vi "FrontPanel.vi"() -> ()   [LabVIEW 2019]
doc: "This VI controls the blindpanel type GHS-2T-1T-700 for a CryoFree DR. Automatization control is embedded in the blindpanel. Keys can be manipulated from within this VI."
uses:
  shared/Inst.FP/Inst.FP.lvclass
  C:/Program Files (x86)/National Instruments/LabVIEW 2019/user.lib/LevyLab/Instrument Framework/SMOs/Instrument/Instrument.lvclass
  C:/Program Files (x86)/National Instruments/LabVIEW 2019/vi.lib/JKI/JKI SMO/SMO/SMO.lvclass
  shared/Inst.FP/Inst.FP.lvclass/Inst.FP.ctl
  shared/Inst.FP/Typedefs/Inst.FP.Push Button--Cluster.ctl
  shared/Inst.FP/Typedefs/Inst.FP.Buttons--Enum.ctl
  <vilib>/Utility/miscctls.llb/LVPointTypeDef.ctl
  ed5445fe-83d3-41b3-b8c0-c155526a2bd6.vi
  <vilib>/JDP Science/JSONtext/JSON text to Variant.vi
  Lib/Lib.llb/ErrCodeStatusLkup.vi
  <vilib>/JDP Science/JSONtext/LVClass Serializer/JSONtext LVClass Serializer.lvclass
  Lib/Lib.llb/Pfeiffer Vacuum.lvlib
  Lib/Lib.llb/MView.lvlib
  Lib/Lib.llb/Busy PopUp.lvlib
  <userlib>/LevyLab/Instrument Framework/SMOs/Instrument/Instrument.lvclass
  <vilib>/JKI/JKI SMO/SMO/SMO.lvclass
panel:
  in  "Inst.FP":refnum<class "Inst.FP.lvclass">
  out "VIRef":T1 {"Array DataType" format="%.0x"; "WaveForm Type" format="%.0x"; "RefNum Type" format="%.0x"; "DataType" format="%.0x"}
  out "ControlNames":string[](array[string])
  in  "Toolbar Panel":enum32{"Page 1", "Page 2"}(tab)
  in  "Load config":bool
  in  "Save config":bool
  in  "Start":bool
  in  "Stop":bool
  out "VI Version":string caption="V"
  out "PT2.Data Array":dbl[](array[numeric])
  in  "Error panel":enum32{"Page 1"}(tab)
  out "PT2.Error":errorcluster
  out "MG.Error":errorcluster
  out "PT1.Error":errorcluster
  out "GHS.Error":errorcluster
  out "PT1.Data Array":dbl[](array[numeric])
  in  "Main Panel":enum32{"Page 1"}(tab)
  out "GHS.P Cluster":T2 {"P1" format="%.1f"; "P2" format="%.1f"; "P3" format="%.1f"; "P4" format="%.1f"; "P5" format="%.1f"; "P6" format="%.1f"; "P7" format="%.1f"; "Flow" format="%#_4f"; "Pstill (P8)" format="%.1e"}
  out "GHS.Alarm?":bool caption="Alarm"
  in  "Main Panel Tabs":T3(tab)
  out "GHS.Layout2.Label1":string
  out "GHS.Layout2.Label2":string
  out "GHS.Layout1.Label1":string
  out "GHS.Layout1.Label2":string
  out "GHS.Mode":u16(ring) items=["AUTO MODE OFF", "START", "CONDENSING 3He", "CONDENSING 4He", "NORMAL CIRCULATION", "RECOVERY OF THE MIXTURE", "RECOVERY: BLOCKAGE OR OVERPRESSURE"]
  out "GHS.Flow":sgl caption="FLOW" format="%#_3f"
  out "GHS.P5":sgl caption="P5"
  out "GHS.P4":sgl caption="P4"
  out "GHS.P3":sgl caption="P3"
  out "GHS.P1":sgl caption="P1"
  out "GHS.P2":sgl caption="P2"
  out "GHS.P7":sgl(slide) caption="3He" min=0 max=2 scale=0.0..2000.0 scale format="%.2f"
  out "GHS.P6":sgl(slide) caption="4He" min=0 max=2 scale=0.0..2000.0 scale format="%.2f"
  out "GHS.Panel ID":string
  in  "GHS Layout Panel":enum32{"OLD", "NEW"}(tab)
  in  "GHS.Layout1.Buttons":T4
  out "GHS.Layout1.LEDs":T5
  in  "GHS.Layout2.Buttons":T4
  out "GHS.Layout2.LEDs":T6
  out "GHS.PC":sgl caption="PC"
  in  "Tab Control 2":enum32{"Plots", "Error Log"}(tab)
  out "PT2 Pressures Plot":cluster{"Time":dbl[], "Value":dbl[]}[](graph)
  out "PT2.Error Log":string[][](table)
  in  "PT2.Start":bool
  in  "PT2.Stop":bool
  in  "PT2.ResetValues":bool
  out "PT2.Error Code":i32 caption="PT Error Code"
  out "PT2.Error Text":string="NO ERROR" caption="PT Error"
  out "PT2.P High":cluster{dbl, dbl, dbl, dbl}(slide) caption="P High" scale=150.0..450.0
  out "PT2.P Low":cluster{dbl, dbl, dbl, dbl}(slide) caption="P Low" scale=0.0..300.0
  out "PT2.P Avg":cluster{"Low":dbl, "High":dbl} caption="P Avg"
  out "PT2.Helium":cluster{dbl, dbl, dbl, dbl}(slide) caption="Helium" scale=0.0..95.0
  out "PT2.Water In":cluster{dbl, dbl, dbl, dbl}(slide) caption="Water In" scale=0.0..35.0
  out "PT2.Water Out":cluster{dbl, dbl, dbl, dbl}(slide) caption="Water Out" scale=0.0..60.0
  out "PT2.State":u16(ring) caption="PT Status" items=["Compressor OFF", "Compressor ON", ""]
  out "PT2.Motor":cluster{dbl, dbl}(slide) caption="Motor" scale=0.0..30.0
  out "PT2.Oil":cluster{dbl, dbl, dbl, dbl}(slide) caption="Oil" scale=0.0..60.0
  out "PT1.P Low":cluster{dbl, dbl, dbl, dbl}(slide) caption="P Low" scale=0.0..300.0
  out "PT1.P High":cluster{dbl, dbl, dbl, dbl}(slide) caption="P High" scale=150.0..450.0
  out "PT1.P Avg":cluster{"Low":dbl, "High":dbl} caption="P Avg"
  out "PT1.Motor":cluster{dbl, dbl}(slide) caption="Motor" scale=0.0..30.0
  out "PT1.Oil":cluster{dbl, dbl, dbl, dbl}(slide) caption="Oil" scale=0.0..60.0
  out "PT1.Helium":cluster{dbl, dbl, dbl, dbl}(slide) caption="Helium" scale=0.0..95.0
  out "PT1.Water Out":cluster{dbl, dbl, dbl, dbl}(slide) caption="Water Out" scale=0.0..60.0
  out "PT1.Water In":cluster{dbl, dbl, dbl, dbl}(slide) caption="Water In" scale=0.0..35.0
  out "PT1.Error Code":i32 caption="PT Error Code"
  out "PT1.Error Text":string="NO ERROR" caption="PT Error"
  in  "PT1.ResetValues":bool
  in  "PT1.Start":bool
  in  "PT1.Stop":bool
  out "PT1.State":u16(ring) caption="PT Status" items=["Compressor OFF", "Compressor ON", ""]
  in  "Tab Control":enum32{"Plots", "Error Log"}(tab)
  out "PT1 Pressures Plot":cluster{"Time":dbl[], "Value":dbl[]}[](graph)
  out "PT1.Error Log":string[][](table)
  out "MG Pressures Plot":cluster{"Time":dbl[], "Value":dbl[]}[](graph)
  out "GHS Pressures Plot":cluster{"Time":dbl[], "Value":dbl[]}[](graph)
  in  "Hide Side Panel":bool
  out "_PT2Port":u16
  out "_PT1Port":u16
  out "_MGPort":refnum<visa-resource-name>="COM4" caption="Port number"
  out "_GHSPort":refnum<visa-resource-name>="COM3" caption="Port number"
  out "_ForceSaveData":bool
  in  "GHS.Button":u8
  out "_SetControl":T7
  in  "S2":enum32{"Page 1"}(tab)
  in  "S2:Reset Error":bool
  in  "S1":enum32{"Page 1"}(tab)
  in  "S1:Reset Error":bool
  out "Curent Log Path":path
  in  "Side Panel":enum32{"Main", "Settings", "Advanced"}(tab)=enum."Settings"
  out "MG.ID String":string caption="ID"
  out "GHS.Response":string caption="Panel response"
  out "MG.Sensors Status":T8={"1"="OK", "2"="OK", "3"="OK", "4"="OK", "5"="OK", "6"="OK"}
  in  "GHS.ADC scaling":T9={"P1"=2500.0, "P2"=2500.0, "P3"=2500.0, "P4"=2500.0, "P5"=2500.0, "P6"=2500.0, "P7"=2500.0, "Flow meter"=682.0, "PC"=10000.0} caption="Front panel ADC scaling factors" {"Flow meter" format="%#.4f"}
  in  "GHS.REC Settings":T10={"P6 low"=20, "P6 high"=1000, "P7 low"=20}
  in  "GHS.NCP5B Settings":cluster{"P6 low":u16}={"P6 low"=20}
  in  "GHS.NCP5 Settings":T10={"P6 low"=20, "P6 high"=1000, "P7 low"=20}
  in  "GHS.S1&2 Settings":cluster{"Enum":enum16{"OFF", "ON"}}
  in  "GHS.P5 Settings":cluster{"P6 low":u16, "P6 high":u16}={"P6 low"=20, "P6 high"=1000}
  out "GHS.REC limits":T11={"P5 warn"=20, "P5 rec"=20, "P5 res"=20}
  out "GHS.NCP5B limits":cluster{"P5 NC4":u16}={"P5 NC4"=20}
  out "GHS.NCP5 limits":T12={"P5 NC1"=20, "P5 NC2"=20, "P5 NC3"=20}
  out "GHS.S1&2 limits":cluster{"S1&S2":enum16{"OFF", "ON"}}
  out "GHS.P5 limits":cluster{"P5 C1":u16, "P5 C2":u16}={"P5 C1"=20, "P5 C2"=20}
  in  "GHS.P6&7 Settings":T13={"P6 low"=20, "P6 high"=1600, "P7 low"=20, "P7 high"=1610}
  out "GHS.P6&7 Limits":T13={"P6 low"=20, "P6 high"=20, "P7 low"=20, "P7 high"=20}
  in  "GHS.Set Values":bool caption="SET VALUES"
  out "MG.Pressures":T14 {"1" format="%-7.2e mbar"; "2" format="%-7.2e mbar"; "3" format="%-7.2e mbar"; "4" format="%-7.2e mbar"; "5" format="%-7.2e mbar"; "6" format="%-7.2e mbar"}
  out "MG.Channel Names":T8={"1"="\"\"", "2"="", "3"="", "4"="", "5"="", "6"=""}
  out "String":string
  in  "Logging Settings":T15={"Plot Data?"=TRUE, "Data Plot Interval"=1.0, "Save Data?"=TRUE, "Data Save Interval"=1.0, "Log Files Folder"=path "C:/LC Data/Data", "Log File Name"="logFP", "Filename Suffix"="_%Y-%m-%d-%H-%M-%S", "New File Interval"=7, "Interval Units"=enum."Days", "Date Format"="%Y-%m-%d %H:%M:%S", "Averages"=4} caption="Data Logging \nOptions" {"Data Save Interval" format="%#_g min"; "Data Plot Interval" format="%#_g min"}
  in  "Hardware Settings":T16={"GHS Port"="COM3", "MG Port"="COM4", "PT1.Enabled?"=FALSE, "MG P8 Channel"=65535, "MG End Recovery?"=FALSE, "PT1 Port"="COM2", "MG Enabled?"=TRUE, "PT1 Address"=16, "S1 Enabled?"=FALSE, "S1 port"="COM2", "S2 Enabled?"=FALSE, "S2 port"="COM2", "Device address S1"=1, "Device address S2"=2, "PT1 Bauds"=115200, "PT2.Enabled?"=FALSE, "PT2 Port"="COM2", "PT2 Address"=16, "PT2 Bauds"=115200, "GHS Bauds"=9600} {"PT2 Address" min=16 max=126 step=1; "MG P8 Channel" items=["Channel 1", "Channel 2", "Channel 3", "Channel 4", "Channel 5", "Channel 6"]; "PT1 Address" min=16 max=126 step=1}
  in  "Automode Settings":T17={"Enable Pressure Check"=FALSE, "Threshold Pressure"=0.0005, "MG Channel"=65535, "Delay Time"=30, "Enable Time Check"=FALSE} {"Delay Time" format="%.0f min"; "MG Channel" items=["Channel 1", "Channel 2", "Channel 3", "Channel 4", "Channel 5", "Channel 6"]; "Threshold Pressure" format="%#_2g mbar"}
  in  "GHS.System Type":enum32{"Wet", "CF"}(radio)=enum."CF" caption="Type"
  in  "GHS.Layout":enum32{"Layout1", "Layout2"}(ring)=enum."Layout2" caption="Panel Layout"
  out "_GHSADCData":dbl[](array[numeric]) caption="Converted ADC Values"
  in  "GHS.Send Command":bool caption="Send"
  out "GHS.Command Response":string
  in  "GHS.Command to Send":string
  out "Automode.Time Reached?":bool
  out "Automode.Pressure Reached?":bool
  out "Automode.Triggered?":bool
  out "Automode.Delay Timer":u32=10 caption="Timer" format="%<%M:%S>t"
  in  "Automode.Start":bool caption="Start"
  out "_VIPath":string caption="VI path"
  out "_GHSRawADCData":i32[](array[numeric]) caption="RAW ADC Values"
  out "MG.Data Array":dbl[](array[numeric]) format="%.3e"
  out "GHS.ADC Data Array":sgl[](array[numeric]) format="%.2f"
  out "GHS.Status Array":u32[](array[numeric])
  # "Error log"
  # "Front panel status"
  # "MaxiGauge status"
  # "Pulse Tube 1 status"
  # "Pulse Tube 2 status"
  # "Leiden Cryogenics"
  # "to \nair"
  # "N.C."
  # "from\novc"
  # "from\nivc"
  # "from still"
  # "to 3He\nin-1"
  # "to 3He\nin-2"
  # "P8"
  # "AUX 1"
  # "BYPASS"
  # "MIXTURE\nCOMPRESSOR"
  # "M2"
  # "P6"
  # "M3"
  # "M1"
  # "AUX PORT-1"
  # "P7"
  # "TRAP"
  # "AUX TRAP"
  # "To \nAir"
  # "From\nIVC"
  # "From Still"
  # "To 3He\nin-1"
  # "To 3He\nin-2"
  # "To \nAir"
  # "N.C."
  # "from\novc"
  # "from\nivc"
  # "from still"
  # "to 3He\nin-1"
  # "to 3He\nin-2"
  # "Leiden Cryogenics"
  # "to \nair"
  # "N.C."
  # "from\novc"
  # "from\nivc"
  # "from still"
  # "to 3He\nin-1"
  # "to 3He\nin-2"
  # "P8"
  # "M2"
  # "P6"
  # "M3"
  # "TRAP"
  # "AUX TRAP"
  # "M1"
  # "AUX PORT-1"
  # "P7"
  # "AUX 1"
  # "To \nAir"
  # "From\nIVC"
  # "From Still"
  # "To 3He\nin-1"
  # "to 3He\nin-1"
  # "To 3He\nin-2"
  # "to \nair"
  # "N.C."
  # "from\novc"
  # "from\nivc"
  # "from still"
  # "to 3He\nin-2"
  # "Pulse Tube 1"
  # "Pulse Tube 2"
  # "Front Panel"
  # "MaxiGauge"
  # "Turbo2 (S2)"
  # "Turbo1 (S1)"
  # "MaxiGauge"
  # "#"
  # "NAME"
  # "PRESSURE"
  # "STATUS"
  # "1"
  # "2"
  # "3"
  # "4"
  # "5"
  # "6"
  # "Automatic mode pressure limits"
  # "Warning: These values influence the operation of the GHS in automatic mode. Please refer to the operation manual and consult with Leiden Cryogenics before changing them."
  # "NAME"
  # "FW"
  # "NEW"
  # "DESCRIPTION"
  # "Stop condensing 4He"
  # "Stop recovering 4He"
  # "Stop condensing 3He"
  # "Stop recovering 3He"
  # "Condensing->open 12"
  # "Condensing->close 9/12"
  # "Condensing->run S1&S2"
  # "NC->open second line"
  # "NC->start MC"
  # "NC->open aux. trap"
  # "NC->stop MC, close 7"
  # "All->P5 alarm"
  # "All->switch to recovery"
  # "All->reset"
  # "Front panel ADC scaling factors"
  # "Data Logging and Plotting"
  # "Front Panel"
  # "MaxiGauge"
  # "Pulse Tube 1"
  # "Pulse Tube 2"
  # "Turbo 1 (S1) (Pfeiffer HiPACE only)"
  # "Turbo2 (S2) (Pfeiffer HiPACE only)"
  # "Automatic condensing"
  # "Send command to Front Panel"
  # "Start condensing when"
  # "and wait"
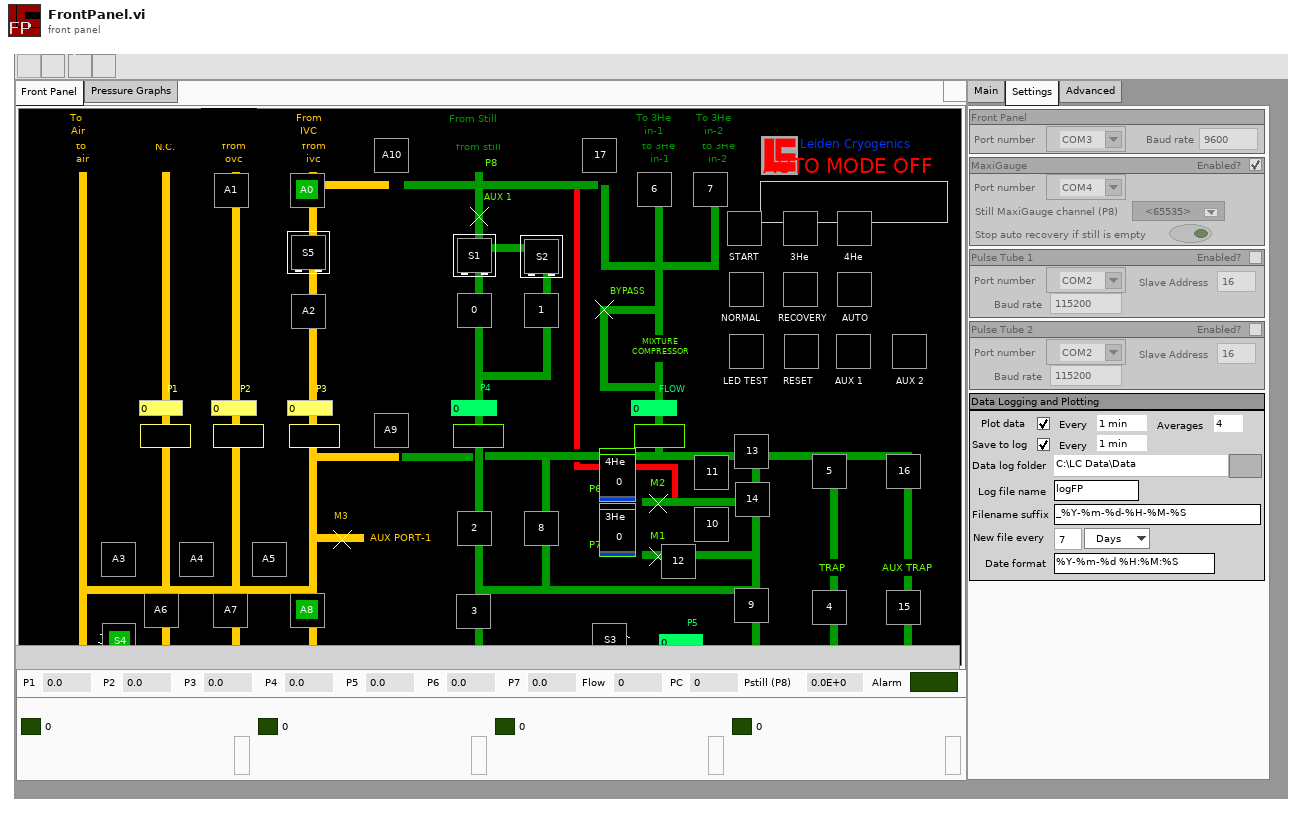
[diagram p1: front panel]
types:
  T1 = cluster{"Control Ref ID":refnum<vi>[], "Full Name":string[], "ClassID":enum16{"<Null>", "1", "2", "Generic", "Decoration", "Text", "Control", "ColorBox", "Boolean", "RefNum", "Variant", "Path", "ListBox", "Table", "Array", "Picture", "ActiveXContainer", "Numeric", "Digital", "NamedNumeric", "ColorRamp", "Slide", "GraphOrChart", "WaveformChart", "WaveformGraph", "IntensityChart", "IntensityGraph", "String", "IOName", "ComboBox", "Cluster", "Panel", "Knob", "NumWithScale", "Ring", "Enum", "GObject", "Plot", "Cursor", "NumericText", "Scale", "ColorScale", "GraphScale", "ColorGraphScale", "TypedRefNum", "OldKnobScale", "MCListbox", "MeasureData", "BVTag", "DAQName", "VISAName", "IVIName", "SlideScale", "TabControl", "Page", "TabArrayTabControl", "ConPane", "57", "58", "59", "60", "61", "62", "63", "64", "SubPanel", "TreeControl", "67", "68", "69", "70", "71", "72", "73", "74", "75", "SplitterBar"}[], "Short Name":string[], "DataType":enum8{"<Null>", "I8", "I16", "I32", "I64", "U8", "U16", "U32", "U64", "SGL", "DBL", "EXT", "CSG", "CDB", "CXT", "0x0F", "0x10", "0x11", "0x12", "0x13", "0x14", "Enum U8", "Enum U16", "Enum U32", "Enum U64", "SGL PQ", "DBL PQ", "EXT PQ", "CSG PQ", "CDB PQ", "CXT PQ", "0x1F", "0x20", "Boolean", "0x22", "0x23", "0x24", "0x25", "0x26", "0x27", "0x28", "0x29", "0x2A", "0x2B", "0x2C", "0x2D", "0x2E", "0x2F", "String", "0x31", "Path", "Pict", "0x34", "0x35", "0x36", "DAQ", "0x38", "0x39", "0x3A", "0x3B", "0x3C", "0x3D", "0x3E", "0x3F", "Array", "0x41", "0x42", "0x43", "0x44", "0x45", "0x46", "0x47", "0x48", "0x49", "0x4A", "0x4B", "0x4C", "0x4D", "0x4E", "0x4F", "Cluster", "0x51", "0x52", "Variant", "Waveform", "0x55", "0x56", "0x57", "0x58", "0x59", "0x5A", "0x5B", "0x5C", "0x5D", "0x5E", "0x5F", "0x60", "0x61", "0x62", "0x63", "0x64", "0x65", "0x66", "0x67", "0x68", "0x69", "0x6A", "0x6B", "0x6C", "0x6D", "0x6E", "0x6F", "Refnum"}[], "RefNum Type":enum8{"Generic", "Datalog File Refnum", "Byte Stream File Refnum", "Device Refnum", "Occurence Refnum", "TCP Connection Refnum", "VISA Refnum (Obsolete)", "Automation Renum", "VI Server Refnum", "Menu Refnum", "IVI Refnum (Obsolete)", "IMAQ Session", "0x0C", "Datasocket Refnum", "VISA Resource", "IVI Logical Name", "UDP Connection Refnum", "Notifier Refnum", "Queue Refnum", "IrDA Refnum", "Hardware Plugin Refnum", "Hardware Plugin Tag Refnum", "DAQmx Refnum", "Event Registration Refnum", ".NET Refnum", "User Event Refnum", "0x1A", "Event Callback", "0x1C", "0x1D", "Only Used Internal to LabVIEW", "Bluetooth", "Data Value References", "RT FIFO", "TDM Streaming"}[], "WaveForm Type":enum8{"<Not a Waveform Type>", "0x01", "Analog 16-bit signed", "Analog Double-Precision", "0x04", "Analog Single Precision", "Timestamp", "Digital Data", "Digital Waveform", "Dynamic Data", "Analog Extended-Precision", "Analog 8-bit unsigned", "Analog 16-bit unsigned", "Analog 32-bit unsigned", "Analog 8-bit signed", "Analog 32-bit signed", "Analog Complex Single-Precision", "Analog Complex Double-Precision", "Analog Complex Extended Precision", "Analog 64-bit signed", "Analog 64-bit unsigned"}[], "Parent":i32[], "Array DataType":enum8{"<Null>", "I8", "I16", "I32", "I64", "U8", "U16", "U32", "U64", "SGL", "DBL", "EXT", "CSG", "CDB", "CXT", "0x0F", "0x10", "0x11", "0x12", "0x13", "0x14", "Enum U8", "Enum U16", "Enum U32", "Enum U64", "SGL PQ", "DBL PQ", "EXT PQ", "CSG PQ", "CDB PQ", "CXT PQ", "0x1F", "0x20", "Boolean", "0x22", "0x23", "0x24", "0x25", "0x26", "0x27", "0x28", "0x29", "0x2A", "0x2B", "0x2C", "0x2D", "0x2E", "0x2F", "String", "0x31", "Path", "Pict", "0x34", "0x35", "0x36", "DAQ", "0x38", "0x39", "0x3A", "0x3B", "0x3C", "0x3D", "0x3E", "0x3F", "Array", "0x41", "0x42", "0x43", "0x44", "0x45", "0x46", "0x47", "0x48", "0x49", "0x4A", "0x4B", "0x4C", "0x4D", "0x4E", "0x4F", "Cluster", "0x51", "0x52", "Variant", "Waveform", "0x55", "0x56", "0x57", "0x58", "0x59", "0x5A", "0x5B", "0x5C", "0x5D", "0x5E", "0x5F", "0x60", "0x61", "0x62", "0x63", "0x64", "0x65", "0x66", "0x67", "0x68", "0x69", "0x6A", "0x6B", "0x6C", "0x6D", "0x6E", "0x6F", "Refnum"}[], "Owning VI":refnum<vi>[], "Active?":bool[]}
  T2 = cluster{"P1":sgl, "P2":sgl, "P3":sgl, "P4":sgl, "P5":sgl, "P6":sgl, "P7":sgl, "Flow":sgl, "PC":sgl, "Pstill (P8)":dbl}
  T3 = enum32{"Front Panel", "PulseTube", "Pressure Graphs"}
  T4 = cluster{"baux2":bool, "bBypass":bool, "b15":bool, "b16":bool, "NC 0":bool, "baux1":bool, "b4":bool, "NC 1":bool, "b5":bool, "breset":bool, "NC 2":bool, "b9":bool, "b14":bool, "NC 3":bool, "b13":bool, "bledtest":bool, "NC 4":bool, "b12":bool, "b10":bool, "NC 5":bool, "b11":bool, "bA0":bool, "NC 9":bool, "b7":bool, "bS3":bool, "NC 12":bool, "b6":bool, "b17":bool, "NC 13":bool, "b8":bool, "b1":bool, "NC 14":bool, "bS2":bool, "b3":bool, "NC 15":bool, "b2":bool, "b0":bool, "NC 16":bool, "bS1":bool, "bA9":bool, "NC 17":bool, "bA8":bool, "bA2":bool, "NC 6":bool, "bs5":bool, "bA10":bool, "NC 7":bool, "bstart":bool, "bA5":bool, "NC 8":bool, "bA7":bool, "bA1":bool, "NC 10":bool, "bauto":bool, "bA4":bool, "NC 11":bool, "bA6":bool, "bS4":bool, "NC 18":bool, "bA3":bool, "b3he":bool, "b4he":bool, "bnorm":bool, "brecov":bool}
  T5 = cluster{"COMPR/AUX 2":bool, "BYPASS":bool, "15":bool, "16":bool, "NC 0":bool, "AUX 1":bool, "4":bool, "NC 1":bool, "5":bool, "RESET":bool, "NC 2":bool, "9":bool, "14":bool, "NC 3":bool, "13":bool, "LED TEST":bool, "NC 4":bool, "12":bool, "10":bool, "NC 5":bool, "11":bool, "A0":bool, "NC 12":bool, "7":bool, "S3":bool, "NC 13":bool, "6":bool, "17":bool, "NC 14":bool, "8":bool, "1":bool, "NC 15":bool, "S2":bool, "3":bool, "NC 16":bool, "2":bool, "0":bool, "NC 17":bool, "S1":bool, "A9":bool, "NC 6":bool, "A8":bool, "A2":bool, "NC 7":bool, "S5":bool, "A10":bool, "NC 8":bool, "START":bool, "A5":bool, "NC 9":bool, "A7":bool, "A1":bool, "NC 10":bool, "AUTO":bool, "A4":bool, "NC 11":bool, "A6":bool, "S4":bool, "NC 18":bool, "A3":bool, "3He":bool, "4He":bool, "NORMAL":bool, "RECOVERY":bool, "PT STATUS":bool}
  T6 = cluster{"COMPR/AUX 2":bool, "BYPASS":bool, "15":bool, "16":bool, "AUX 1":bool, "AUX 1":bool, "4":bool, "AUX 2":bool, "5":bool, "RESET":bool, "AUX 3":bool, "9":bool, "14":bool, "NC 3":bool, "13":bool, "LED TEST":bool, "NC 4":bool, "12":bool, "10":bool, "NC 5":bool, "11":bool, "A0":bool, "NC 12":bool, "7":bool, "S3":bool, "NC 13":bool, "6":bool, "17":bool, "NC 14":bool, "8":bool, "1":bool, "NC 15":bool, "S2":bool, "3":bool, "NC 16":bool, "2":bool, "0":bool, "NC 17":bool, "S1":bool, "A9":bool, "NC 6":bool, "A8":bool, "A2":bool, "NC 7":bool, "S5":bool, "A10":bool, "NC 8":bool, "START":bool, "A5":bool, "NC 9":bool, "A7":bool, "A1":bool, "NC 10":bool, "AUTO":bool, "A4":bool, "NC 11":bool, "A6":bool, "S4":bool, "NC 18":bool, "A3":bool, "3He":bool, "4He":bool, "NORMAL":bool, "RECOVERY":bool, "PT STATUS":bool}
  T7 = cluster{"Name":string, "Scalar":string, "Array":string[][]}
  T8 = cluster{"1":string, "2":string, "3":string, "4":string, "5":string, "6":string}
  T9 = cluster{"P1":dbl, "P2":dbl, "P3":dbl, "P4":dbl, "P5":dbl, "P6":dbl, "P7":dbl, "Flow meter":dbl, "PC":dbl}
  T10 = cluster{"P6 low":u16, "P6 high":u16, "P7 low":u16}
  T11 = cluster{"P5 warn":u16, "P5 rec":u16, "P5 res":u16}
  T12 = cluster{"P5 NC1":u16, "P5 NC2":u16, "P5 NC3":u16}
  T13 = cluster{"P6 low":u16, "P6 high":u16, "P7 low":u16, "P7 high":u16}
  T14 = cluster{"1":dbl, "2":dbl, "3":dbl, "4":dbl, "5":dbl, "6":dbl}
  T15 = cluster{"Plot Data?":bool, "Data Plot Interval":dbl, "Save Data?":bool, "Data Save Interval":dbl, "Log Files Folder":path, "Log File Name":string, "Filename Suffix":string, "New File Interval":u32, "Interval Units":enum16{"Minutes", "Hours", "Days"}, "Date Format":string, "Averages":i32}
  T16 = cluster{"GHS Port":refnum<visa-resource-name>, "MG Port":refnum<visa-resource-name>, "PT1.Enabled?":bool, "MG P8 Channel":u16, "MG End Recovery?":bool, "PT1 Port":refnum<visa-resource-name>, "MG Enabled?":bool, "PT1 Address":u8, "S1 Enabled?":bool, "S1 port":refnum<visa-resource-name>, "S2 Enabled?":bool, "S2 port":refnum<visa-resource-name>, "Device address S1":u8, "Device address S2":u8, "PT1 Bauds":u32, "PT2.Enabled?":bool, "PT2 Port":refnum<visa-resource-name>, "PT2 Address":u8, "PT2 Bauds":u32, "GHS Bauds":u32}
  T17 = cluster{"Enable Pressure Check":bool, "Threshold Pressure":dbl, "MG Channel":u16, "Delay Time":u32, "Enable Time Check":bool}
  T18 = typedef "Inst.FP.lvclass/PublicEvents--Cluster.ctl" = cluster{"MessageFromProcess":refnum<user-event>}
  T19 = cluster{"error":bool, "code":i32, "source":string}
  T20 = cluster{"Dict. Var":u16, "Description":string, "Values":i32[]}[]
  T21 = cluster{"[3]":dbl, "[3]":dbl, "[3]":dbl, "Values[3] 2":dbl}
  T22 = cluster{"[1]":dbl, "[1]":dbl, "[1]":dbl, "Values[1] 2":dbl}
  T23 = cluster{"Values[0]":dbl, "Values[0]":dbl, "Values[0]":dbl, "Values[0] 2":dbl}
  T24 = cluster{"error":bool, "code":i32, "error source":string}
  T25 = cluster{"sensor status info[0]":string, "sensor status info[1]":string, "sensor status info[2]":string, "sensor status info[3]":string, "sensor status info[4]":string, "sensor status info[5]":string}
  T26 = cluster{"Filterred[0]":dbl, "Filterred[1]":dbl, "Filterred[2]":dbl, "Filterred[3]":dbl, "Filterred[4]":dbl, "Filterred[5]":dbl}
  T27 = typedef "Inst.FP.lvclass/Inst.FP.Push Button--Cluster.ctl" = cluster{"Button":T28}
  T28 = typedef "Inst.FP.lvclass/Inst.FP.Buttons--Enum.ctl" = enum16{"Start", "3He", "4He", "Normal", "Recovery", "Auto", "LED Test", "Reset"}
  T29 = cluster{"GHS.ADC Data Array[0]":sgl, "GHS.ADC Data Array[1]":sgl, "GHS.ADC Data Array[2]":sgl, "GHS.ADC Data Array[3]":sgl, "GHS.ADC Data Array[4]":sgl, "GHS.ADC Data Array[5]":sgl, "GHS.ADC Data Array[6]":sgl, "GHS.ADC Data Array[7]":sgl, "GHS.ADC Data Array[8]":sgl}
  T30 = cluster{"GHS.ADC Data Array[0]":sgl, "GHS.ADC Data Array[1]":sgl, "GHS.ADC Data Array[2]":sgl, "GHS.ADC Data Array[3]":sgl, "GHS.ADC Data Array[4]":sgl, "GHS.ADC Data Array[5]":sgl, "GHS.ADC Data Array[6]":sgl, "GHS.ADC Data Array[7]":sgl, "GHS.ADC Data Array[8]":sgl, dbl}
  T31 = enum32{"Page Enabled", "Page Disabled", "Page Disabled & Grayed"}
  T32 = enum32{"invalid app kind", "Development System", "Run Time System", "Student Edition", "Embedded LabVIEW", "Evaluation", "Custom"}
  T33 = cluster{"array of 4 x 16 bit unsigned[0]":u16, "array of 4 x 16 bit unsigned[1]":u16, "array of 4 x 16 bit unsigned[2]":u16, "array of 4 x 16 bit unsigned[3]":u16}
  T34 = cluster{"array of 2 x 16 bit unsigned[0]":u16, "array of 2 x 16 bit unsigned[1]":u16}
  T35 = cluster{"array of 3 x 16 bit unsigned[0]":u16, "array of 3 x 16 bit unsigned[1]":u16, "array of 3 x 16 bit unsigned[2]":u16}
  T36 = cluster{"Array[0]":string, "Array[1]":string, "Array[2]":string, "Array[3]":string, "Array[4]":string, "Array[5]":string}
  T37 = typedef "LVPointTypeDef.ctl" = cluster{"Horizontal":i16, "Vertical":i16}
  T38 = typedef "LVRectTypeDef.ctl" = cluster{"Left":i16, "Top":i16, "Right":i16, "Bottom":i16}
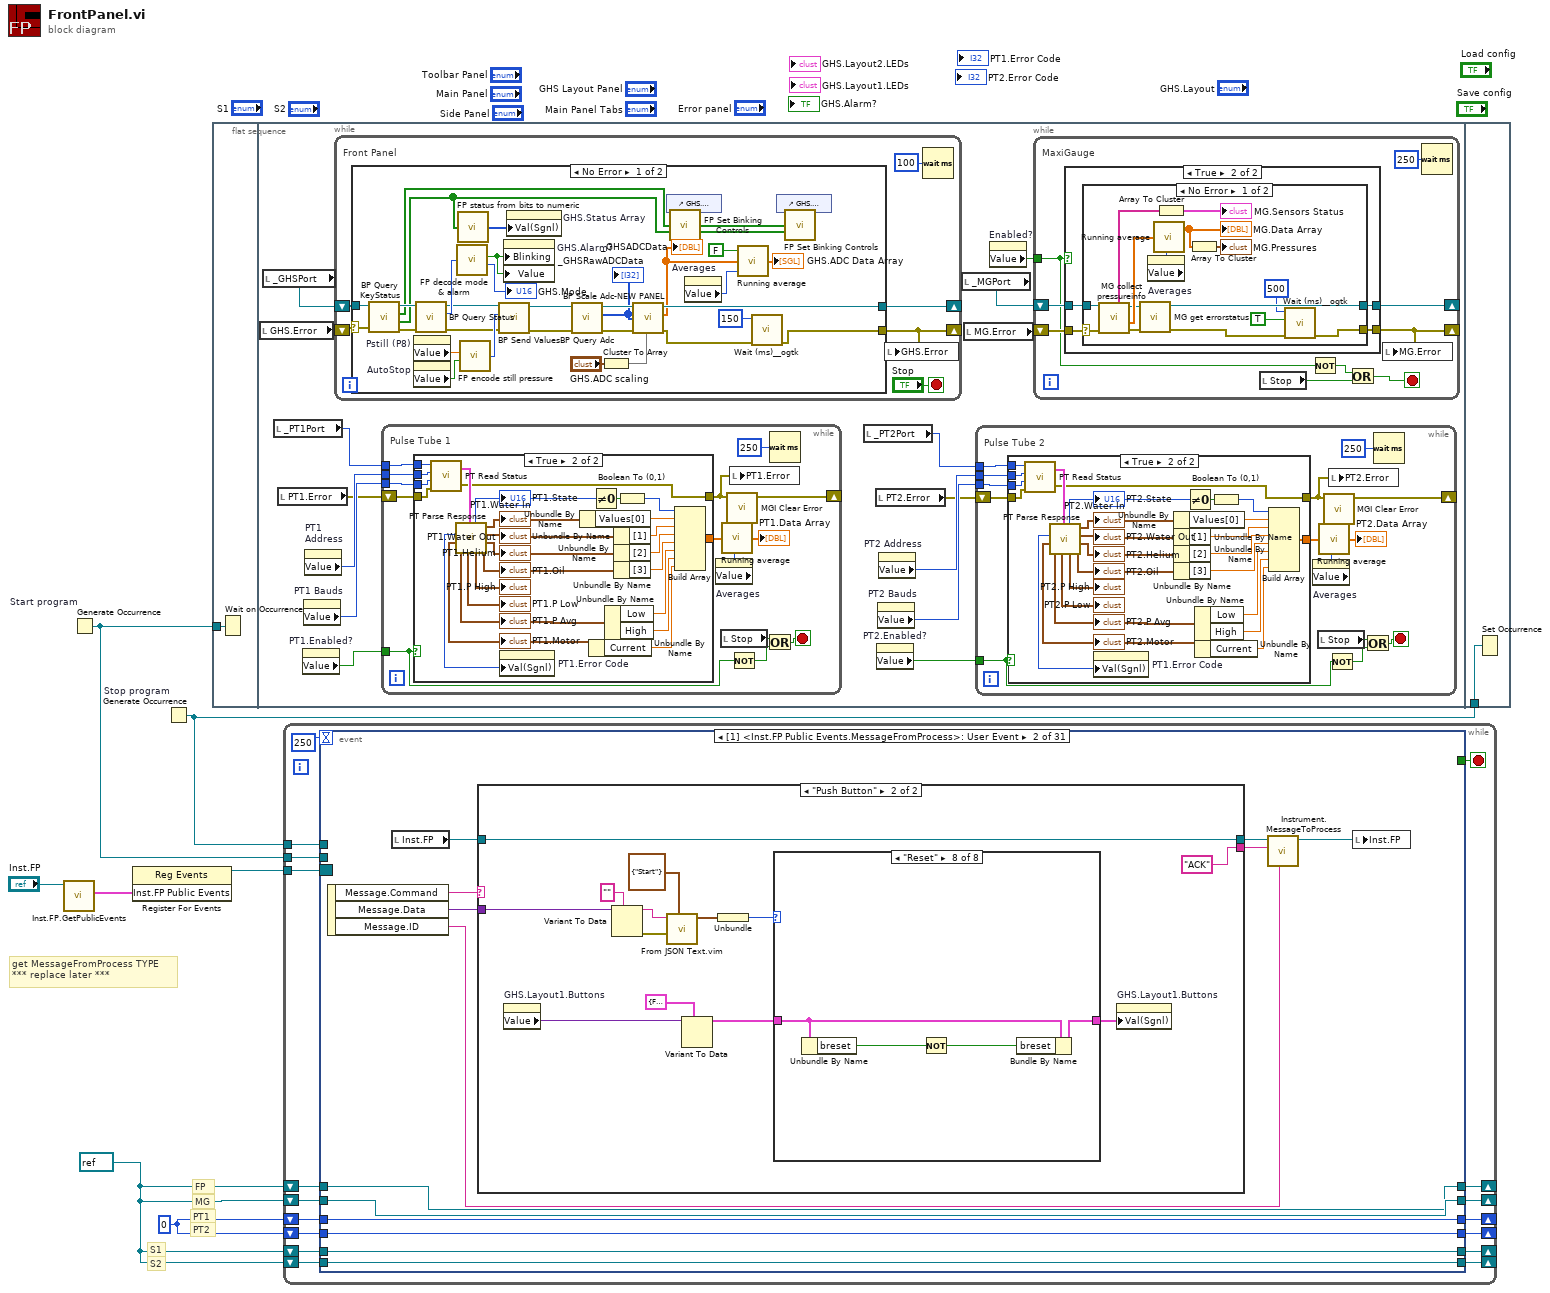
[diagram p0: block diagram]
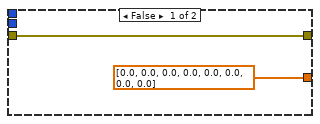
[diagram p2: hidden frame]
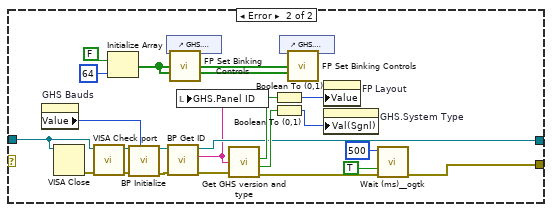
[diagram p3: hidden frame]
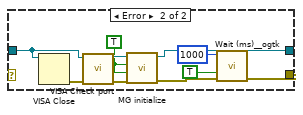
[diagram p5: hidden frame]
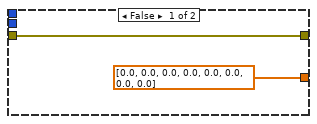
[diagram p6: hidden frame]
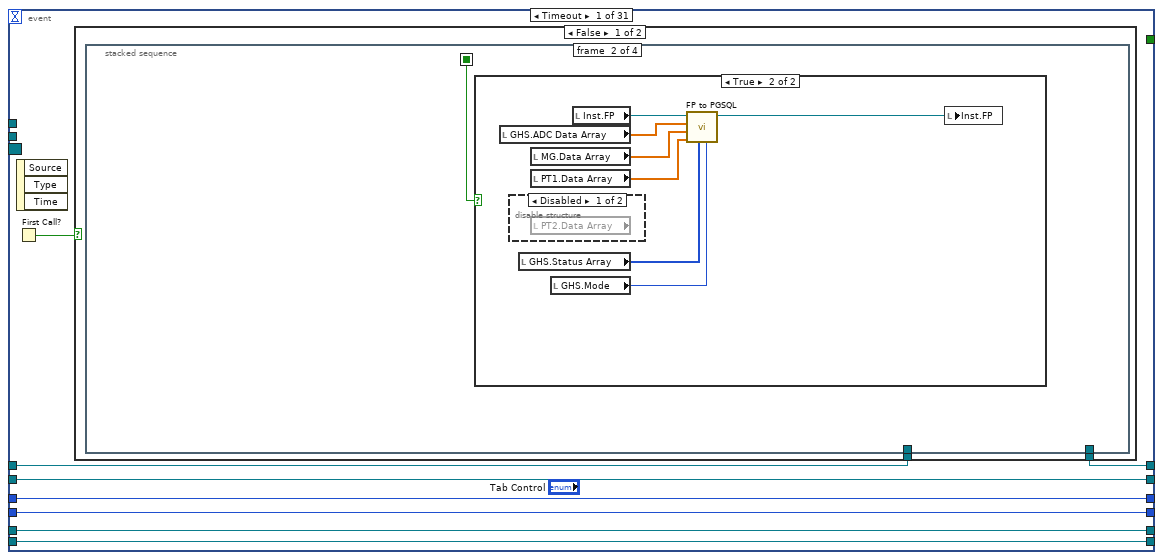
[diagram p7: hidden frame]
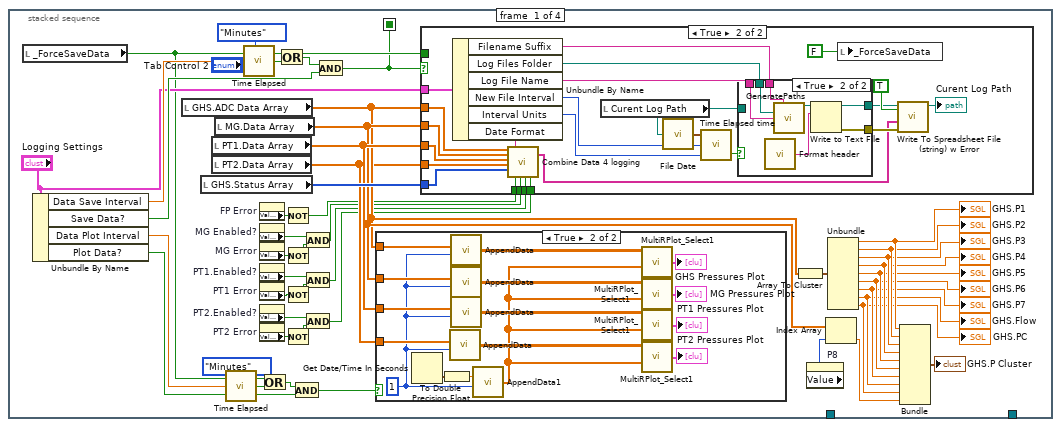
[diagram p8: hidden frame]
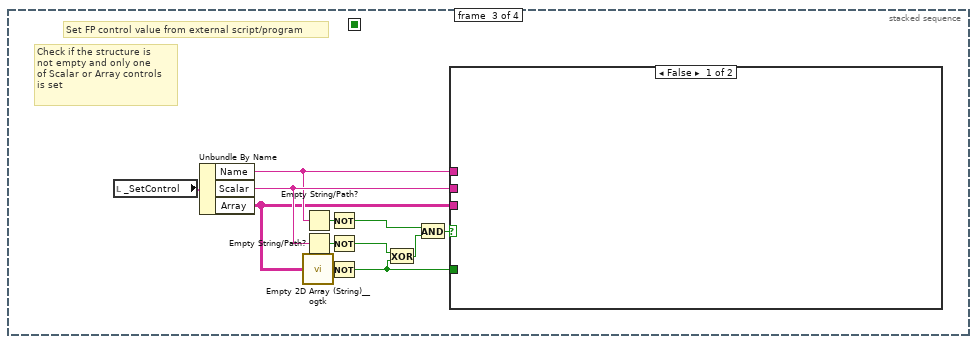
[diagram p14: hidden frame]
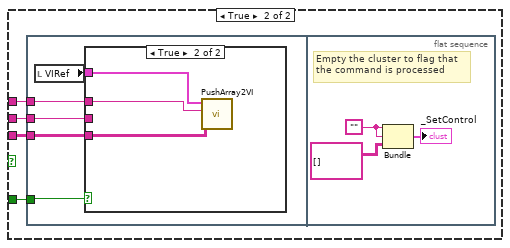
[diagram p15: hidden frame]
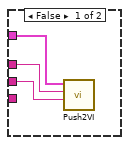
[diagram p16: hidden frame]
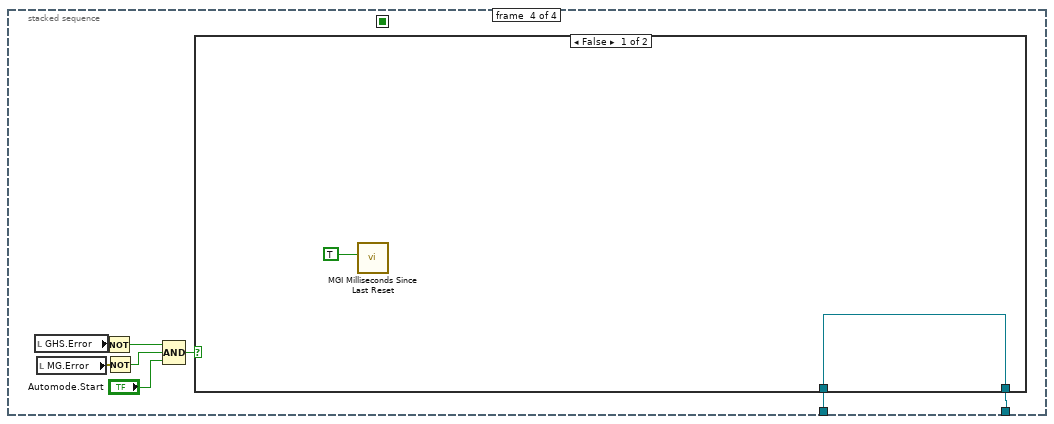
[diagram p17: hidden frame]
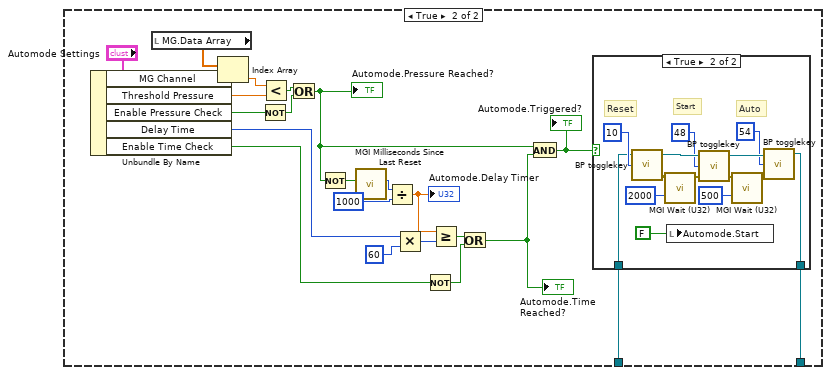
[diagram p18: hidden frame]
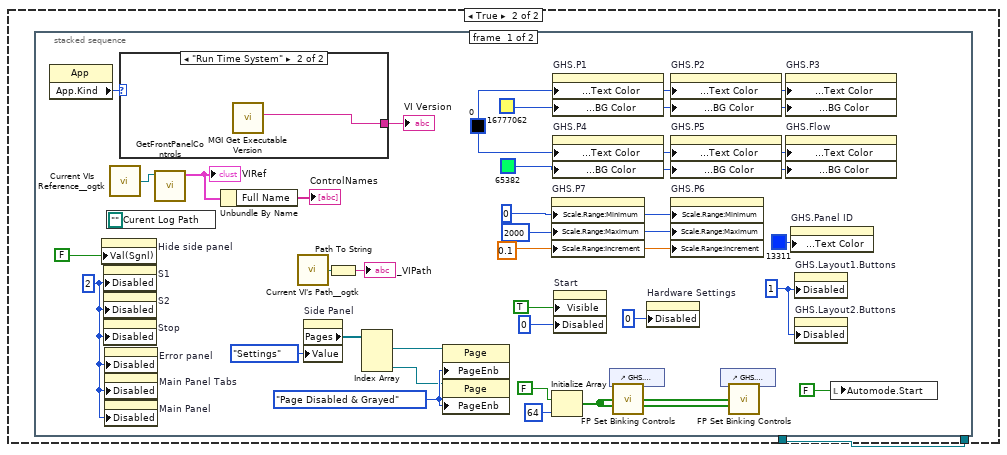
[diagram p20: hidden frame]
diagram:
  w4 = u8 0 ("x+1")
  w5 = refnum<visa-resource-name> refnum ("PT port")
  # "get MessageFromProcess TYPE\n*** replace later ***"
  # "S2"
  # "S1"
  # "MG"
  # "PT1"
  # "PT2"
  # "FP"
  n1 = call "Inst.FP.GetPublicEvents.vi"("Inst.FP in"="Inst.FP") -> ("Inst.FP Public Events"=w2:T18)  [unwired: 8 in, 2 out]
  n2 = Generate Occurrence "Start program"() -> (w7:refnum<k4>)
  n3 = register-events(w2) -> (reference out=w3:refnum<event-registration>)  [unwired: 2 in, 1 out]
  n4 = Generate Occurrence "Stop program"() -> (w6:refnum<k4>)
  n5 = flat-sequence {
    tunnel: w7 -> [w8]
    tunnel: w6 -> [w207]
    frame #0 {
      n6 = Wait on Occurrence(2:w8) -> ()  [unwired: 2 in, 1 out]
    }
    frame #1 {
      n7 = local read "GHS.Error"() -> (w19:errorcluster)
      n8 = local read "_GHSPort"() -> (w14:refnum<visa-resource-name>)
      n9 = local read "_PT1Port"() -> (w10:u16)
      n10 = local read "PT1.Error"() -> (w11:errorcluster)
      n11 = property on="PT1.Enabled?" class="Bool (strict)"() -> ("Value"=w22:bool)  [unwired: 2 in, 2 out]
      n12 = property on="PT1 Bauds" class="DigNum (strict)"() -> ("Value"=w20:u32)  [unwired: 2 in, 2 out]
      n13 = property on="PT1 \nAddress" class="DigNum (strict)"() -> ("Value"=w23:u8)  [unwired: 2 in, 2 out]
      n14 = while {
        shift-right: [w69] -> _
        shift-left: w19 -> [w70]
        shift-right: [w67] -> _
        shift-left: w14 -> [w68]
        stop <- "Stop" stop-if-true
        # "Front Panel"
        n15 = case shown="No Error" w70 {
          selector: w70 -> [w100 _]
          tunnel: [w81 w114] -> w67
          tunnel: [w79 w112] -> w69
          tunnel: w68 -> [w101 w115]
          frame No Error {
            n16 = call "BP Query KeyStatus.vi"("error in"=w100, "FrontPanel port"=w101) -> ("error out"=w89:T19, "Button states"=w72:bool[], "Blinking States"=w73:bool[], "FrontPanel port"=w90:refnum<visa-resource-name>)  [unwired: 2 in]
            n17 = property on="Pstill (P8)" class="DigNum (strict)"() -> ("Value"=w91:dbl)  [unwired: 2 in, 2 out]
            n18 = property on="AutoStop" class="Bool (strict)"() -> ("Value"=w92:bool)  [unwired: 2 in, 2 out]
            n19 = call "BP Query Status.vi"("error in"=w89, "FrontPanel port"=w90) -> ("error out"=w94:T19, "status word (32 bit unsigned)"=w97:u32, "FrontPanel port"=w95:refnum<visa-resource-name>)  [unwired: 3 in]
            n20 = call "FP decode mode & alarm.vi"("status word (32 bit unsigned)"=w97) -> ("Boolean"=w93:bool, "Numeric"=→"GHS.Mode":u32)  [unwired: 4 in]
            n21 = call "FP status from bits to numeric.vi"("FP Status bits"=w72) -> ("FP status number"=w99:u32[])  [unwired: 4 in]
            n22 = call "FP encode still pressure.vi"("Value 2"=w92, "Value"=w91) -> ("Numeric"=w96:u16)  [unwired: 4 in]
            n23 = call "BP Send Values.vi"("error in"=w94, "value to send"=w96, "FrontPanel port"=w95) -> ("error out"=w83:T19, "FrontPanel port"=w84:refnum<visa-resource-name>)  [unwired: 3 in]
            n24 = property on="GHS.Alarm?" class="Bool (strict)"("Blinking"=w93, "Value"=w93) -> ()  [unwired: 2 in, 2 out]
            n25 = property on="GHS.Status Array" class="Arr (strict)"("Val(Sgnl)"=w99) -> ()  [unwired: 2 in, 2 out]
            n26 = call "BP Query Adc.vi"("error in"=w83, "FrontPanel port"=w84) -> ("error out"=w80:T19, "array of 9 x 16 bit signed"=w75:i32[], "FrontPanel port"=w81:refnum<visa-resource-name>)  [unwired: 3 in]
            "_GHSRawADCData" <- w75
            n27 = Cluster To Array(cluster="GHS.ADC scaling") -> (array=w82:dbl[])
            n28 = call "BP Scale Adc-NEW PANEL.vi"("input array scaling factors,8(9) x 16 bit uint"=w82, "input array 8(9) x 16bit uint"=w75) -> ("output array 8(9) x single prec. incl flow"=w74:sgl[])  [unwired: 4 in, 1 out]
            "_GHSADCData" <- w74
            n29 = control-ref of="GHS.Layout1.LEDs"() -> (w77:refnum<vi>)
            n30 = call "FP Set Binking Controls.vi"("Cluster in"=w77, "Array of blinking states"=w73, "Array of relais states"=w72) -> ()  [unwired: 13 in]
            n31 = property on="Averages" class="DigNum (strict)"() -> ("Value"=w88:i32)  [unwired: 2 in, 2 out]
            n32 = call "Running average.vi"("Window Size"=w88, "New values"=w74, "Filter Zeroes? (T)"=FALSE) -> ("Filterred"=→"GHS.ADC Data Array":dbl[])  [unwired: 1 in]
            n33 = call <userlib>:"Wait (ms)__ogtk.vi"("error in (no error)"=w80, "milliseconds to wait"=u32 150) -> ("error out"=w79:errorcluster)  [unwired: 8 in, 1 out]
            n34 = control-ref of="GHS.Layout2.LEDs"() -> (w76:refnum<vi>)
            n35 = call "FP Set Binking Controls.vi"("Cluster in"=w76, "Array of blinking states"=w73, "Array of relais states"=w72) -> ()  [unwired: 13 in]
          }
          frame Error {
            n36 = property on="GHS Bauds" class="DigNum (strict)"() -> ("Value"=w107:u32)  [unwired: 2 in, 2 out]
            n37 = VISA Close(VISA resource name=w115) -> (error out=w124:errorcluster)  [unwired: 1 in]
            n38 = call "VISA Check port.vi"("error in (no error)"=w124, "VISA Resource Name in"=w115) -> ("error out"=w123:errorcluster, "VISA Resource Name out"=w122:refnum<visa-resource-name>)  [unwired: 8 in]
            n39 = Initialize Array(FALSE, 64 ("dimension size")) -> (w102:bool[])
            n40 = call "BP Initialize.vi"("FP baud rate"=w107, "error in (no error)"=w123, "FrontPanel port"=w122) -> ("error out"=w121:errorcluster, "FrontPanel port"=w120:refnum<visa-resource-name>)  [unwired: 4 in]
            n41 = control-ref of="GHS.Layout1.LEDs"() -> (w104:refnum<vi>)
            n42 = call "BP Get ID.vi"("error in (no error)"=w121, "FrontPanel port"=w120) -> ("error out"=w109:errorcluster, "Device ID string"=w113:string, "FrontPanel port"=w114:refnum<visa-resource-name>)  [unwired: 6 in, 1 out]
            n43 = call "FP Set Binking Controls.vi"("Cluster in"=w104, "Array of blinking states"=w102, "Array of relais states"=w102) -> ()  [unwired: 13 in]
            n44 = local write "GHS.Panel ID"(w113) -> ()
            n45 = call "Get GHS version and type.vi"("ID string"=w113, "error in (no error)"=w109) -> ("Panel Version"=w116:bool, "System Type"=w118:bool, "error out"=w108:errorcluster)  [unwired: 4 in]
            n46 = Boolean To (0,1)(Boolean=w116) -> (0, 1=w117:i16)
            n47 = Boolean To (0,1)(Boolean=w118) -> (0, 1=w119:i16)
            n48 = control-ref of="GHS.Layout2.LEDs"() -> (w103:refnum<vi>)
            n49 = call "FP Set Binking Controls.vi"("Cluster in"=w103, "Array of blinking states"=w102, "Array of relais states"=w102) -> ()  [unwired: 13 in]
            n50 = property on="FP Layout" class="TabCtl (strict)"("Value"=w117) -> ()  [unwired: 2 in, 2 out]
            n51 = property on="GHS.System Type" class="RadioBtnsControl (strict)"("Val(Sgnl)"=w119) -> ()  [unwired: 2 in, 2 out]
            n52 = call <userlib>:"Wait (ms)__ogtk.vi"("error in (no error)"=w108, "Wait on Error (FALSE)"=TRUE, "milliseconds to wait"=u32 500) -> ("error out"=w112:errorcluster)  [unwired: 7 in, 1 out]
          }
        }
        n53 = local write "GHS.Error"(w69) -> ()
        n54 = Wait (ms)(milliseconds to wait=u32 100) -> ()  [unwired: 1 out]
      }
      n55 = while {
        tunnel: w10 -> [w177]
        tunnel: w23 -> [w176]
        tunnel: w22 -> [w167]
        tunnel: w20 -> [w173]
        shift-right: [w166] -> _
        shift-left: w11 -> [w172]
        stop <- w170 stop-if-true
        # "Pulse Tube 1"
        n56 = case shown="True" w167 {
          tunnel: [dbl[] [0.0, 0.0, 0.0, 0.0, 0.0, 0.0, 0.0, 0.0] w194] -> w178
          tunnel: w177 -> [_ w193]
          tunnel: w172 -> [w179 w192]
          tunnel: w176 -> [_ w191]
          tunnel: w173 -> [_ w186]
          tunnel: [w179 w185] -> w165
          frame False {
          }
          frame True {
            n57 = call "PT Read Status.vi"("error in (no error)"=w192, "Baud"=w186, "Slave Address"=w191, "Com Port #"=w193) -> ("error out"=w185:errorcluster, "Response"=w195:T20)
            n58 = call "PT Parse Response.vi"("Response"=w195) -> ("Oil temp"=w200:T21, "He temp"=w199:cluster{"[2]":dbl, "[2]":dbl, "[2]":dbl, dbl}, "Out water temp"=w198:T22, "In water temp"=w197:T23, "P_high"=→"PT1.P High":cluster{"[0]":dbl, "[0]":dbl, "[0]":dbl, dbl}, "Numeric"=w204:i32, "P_low"=→"PT1.P Low":cluster{"[1]":dbl, "[1]":dbl, "[1]":dbl, dbl}, "Average pressure"=w190:cluster{"Low":dbl, "High":dbl}, "Current"=w184:cluster{"Current":dbl, "Threshold":dbl}, "PT Error"=w196:i32)  [unwired: 1 in]
            "PT1.Oil" <- w200
            "PT1.Motor" <- w184
            "PT1.State" <- w204
            "PT1.Water Out" <- w198
            "PT1.Water In" <- w197
            "PT1.Helium" <- w199
            "PT1.P Avg" <- w190
            n59 = property on="PT1.Error Code" class="DigNum (strict)"("Val(Sgnl)"=w196) -> ()  [unwired: 2 in, 2 out]
            n60 = Unbundle By Name(w197) -> ("Values[0]"=w187:dbl)
            n61 = Unbundle By Name(w184) -> ("Current"=w183:dbl)
            n62 = Not Equal To 0?(x=w204) -> (x != 0?=w205:bool)
            n63 = Unbundle By Name(w190) -> ("Low"=w189:dbl, "High"=w188:dbl)
            n64 = Unbundle By Name(w198) -> ("[1]"=w203:dbl)
            n65 = Unbundle By Name(w199) -> ("[2]"=w202:dbl)
            n66 = Unbundle By Name(w200) -> ("[3]"=w201:dbl)
            n67 = Boolean To (0,1)(Boolean=w205) -> (0, 1=w206:i16)
            n68 = Build Array(w206, w187, w203, w202, w201, w189, w188, w183) -> (w194:dbl[])
          }
        }
        n69 = property on="Averages" class="DigNum (strict)"() -> ("Value"=w175:i32)  [unwired: 2 in, 2 out]
        n70 = local read "Stop"() -> (w169:bool)
        n71 = call "Running average.vi"("Window Size"=w175, "New values"=w178) -> ("Filterred"=→"PT1.Data Array":dbl[])  [unwired: 2 in]
        n72 = call <userlib>:"MGI Clear Error.vi"("Error In"=w165) -> ("Error Out"=w166:errorcluster)  [unwired: 6 in]
        n73 = Not(x=w167) -> (.not. x?=w168:bool)
        n74 = local write "PT1.Error"(w165) -> ()
        n75 = Or(x=w169, y=w168) -> (x .or. y?=w170:bool)
        n76 = Wait (ms)(milliseconds to wait=u32 250) -> ()  [unwired: 1 out]
      }
      n77 = local read "_PT2Port"() -> (w9:u16)
      n78 = local read "PT2.Error"() -> (w12:errorcluster)
      n79 = property on="PT2.Enabled?" class="Bool (strict)"() -> ("Value"=w16:bool)  [unwired: 2 in, 2 out]
      n80 = property on="PT2 Bauds" class="DigNum (strict)"() -> ("Value"=w15:u32)  [unwired: 2 in, 2 out]
      n81 = property on="PT2 Address" class="DigNum (strict)"() -> ("Value"=w17:u8)  [unwired: 2 in, 2 out]
      n82 = local read "_MGPort"() -> (w13:refnum<visa-resource-name>)
      n83 = local read "MG.Error"() -> (w18:errorcluster)
      n84 = while {
        tunnel: w9 -> [w36]
        tunnel: w17 -> [w35]
        tunnel: w16 -> [w26]
        tunnel: w15 -> [w32]
        shift-right: [w25] -> _
        shift-left: w12 -> [w31]
        stop <- w29 stop-if-true
        # "Pulse Tube 2"
        n85 = case shown="True" w26 {
          tunnel: [dbl[] [0.0, 0.0, 0.0, 0.0, 0.0, 0.0, 0.0, 0.0] w53] -> w37
          tunnel: w36 -> [_ w52]
          tunnel: w31 -> [w38 w51]
          tunnel: w35 -> [_ w50]
          tunnel: w32 -> [_ w45]
          tunnel: [w38 w44] -> w24
          frame False {
          }
          frame True {
            n86 = call "PT Read Status.vi"("error in (no error)"=w51, "Baud"=w45, "Slave Address"=w50, "Com Port #"=w52) -> ("error out"=w44:errorcluster, "Response"=w54:T20)
            n87 = call "PT Parse Response.vi"("Response"=w54) -> ("Oil temp"=w59:T21, "He temp"=w58:cluster{"[2]":dbl, "[2]":dbl, "[2]":dbl, dbl}, "Out water temp"=w57:T22, "In water temp"=w56:T23, "P_high"=→"PT2.P High":cluster{"[0]":dbl, "[0]":dbl, "[0]":dbl, dbl}, "Numeric"=w63:i32, "P_low"=→"PT2.P Low":cluster{"[1]":dbl, "[1]":dbl, "[1]":dbl, dbl}, "Average pressure"=w49:cluster{"Low":dbl, "High":dbl}, "Current"=w43:cluster{"Current":dbl, "Threshold":dbl}, "PT Error"=w55:i32)  [unwired: 1 in]
            "PT2.Oil" <- w59
            "PT2.Motor" <- w43
            "PT2.State" <- w63
            "PT2.Water Out" <- w57
            "PT2.Water In" <- w56
            "PT2.Helium" <- w58
            "PT2.P Avg" <- w49
            n88 = property on="PT1.Error Code" class="DigNum (strict)"("Val(Sgnl)"=w55) -> ()  [unwired: 2 in, 2 out]
            n89 = Unbundle By Name(w56) -> ("Values[0]"=w46:dbl)
            n90 = Unbundle By Name(w57) -> ("[1]"=w62:dbl)
            n91 = Unbundle By Name(w58) -> ("[2]"=w61:dbl)
            n92 = Unbundle By Name(w59) -> ("[3]"=w60:dbl)
            n93 = Not Equal To 0?(x=w63) -> (x != 0?=w64:bool)
            n94 = Unbundle By Name(w49) -> ("Low"=w48:dbl, "High"=w47:dbl)
            n95 = Unbundle By Name(w43) -> ("Current"=w42:dbl)
            n96 = Boolean To (0,1)(Boolean=w64) -> (0, 1=w65:i16)
            n97 = Build Array(w65, w46, w62, w61, w60, w48, w47, w42) -> (w53:dbl[])
          }
        }
        n98 = property on="Averages" class="DigNum (strict)"() -> ("Value"=w34:i32)  [unwired: 2 in, 2 out]
        n99 = local read "Stop"() -> (w28:bool)
        n100 = call "Running average.vi"("Window Size"=w34, "New values"=w37) -> ("Filterred"=→"PT2.Data Array":dbl[])  [unwired: 2 in]
        n101 = call <userlib>:"MGI Clear Error.vi"("Error In"=w24) -> ("Error Out"=w25:errorcluster)  [unwired: 6 in]
        n102 = Not(x=w26) -> (.not. x?=w27:bool)
        n103 = local write "PT2.Error"(w24) -> ()
        n104 = Or(x=w28, y=w27) -> (x .or. y?=w29:bool)
        n105 = Wait (ms)(milliseconds to wait=u32 250) -> ()  [unwired: 1 out]
      }
      n106 = property on="Enabled?" class="Bool (strict)"() -> ("Value"=w21:bool)  [unwired: 2 in, 2 out]
      n107 = while {
        tunnel: w21 -> [w126]
        shift-right: [w130] -> _
        shift-left: w18 -> [w129]
        shift-right: [w128] -> _
        shift-left: w13 -> [w131]
        stop <- w127 stop-if-true
        # "MaxiGauge"
        n108 = case shown="True" w126 {
          tunnel: w131 -> [w135 w139]
          tunnel: [w134 w138] -> w130
          tunnel: w129 -> [w134 w137]
          tunnel: [w135 w136] -> w128
          frame False {
          }
          frame True {
            n109 = case shown="No Error" w137 {
              selector: w137 -> [w146 _]
              tunnel: w139 -> [w154 w164]
              tunnel: [w140 w155] -> w138
              tunnel: [w153 w163] -> w136
              frame No Error {
                n110 = call "MG collect pressureinfo.vi"("error in"=w146, "MaxiGauge port"=w154) -> ("error out"=w151:T24, "sensor values"=w149:dbl[], "MaxiGauge port"=w145:refnum<visa-resource-name>, "sensor status info"=w144:string[])  [unwired: 4 in, 2 out]
                n111 = call "MG get errorstatus.vi"("error in"=w151, "MaxiGauge port"=w145) -> ("error out"=w141:T24, "MaxiGauge port"=w153:refnum<visa-resource-name>)  [unwired: 2 in, 2 out]
                n112 = property on="Averages" class="DigNum (strict)"() -> ("Value"=w148:i32)  [unwired: 2 in, 2 out]
                n113 = call "Running average.vi"("Window Size"=w148, "New values"=w149) -> ("Filterred"=w147:dbl[])  [unwired: 2 in]
                "MG.Data Array" <- w147
                n114 = Array To Cluster(array=w144) -> (cluster=→"MG.Sensors Status":T25)
                n115 = Array To Cluster(array=w147) -> (cluster=→"MG.Pressures":T26)
                n116 = call <userlib>:"Wait (ms)__ogtk.vi"("error in (no error)"=w141, "Wait on Error (FALSE)"=TRUE, "milliseconds to wait"=u32 500) -> ("error out"=w140:errorcluster)  [unwired: 7 in, 1 out]
              }
              frame Error {
                w159 = TRUE ("ID query")
                n117 = VISA Close(VISA resource name=w164) -> (error out=w162:errorcluster)  [unwired: 1 in]
                n118 = call "VISA Check port.vi"("error in (no error)"=w162, "VISA Resource Name in"=w164) -> ("error out"=w161:errorcluster, "VISA Resource Name out"=w160:refnum<visa-resource-name>)  [unwired: 8 in]
                n119 = call "MG initialize.vi"("error in (no error)"=w161, "MG query errorstatus"=w159, "ID query"=w159, "MaxiGauge port"=w160) -> ("error out"=w156:errorcluster, "MaxiGauge port"=w163:refnum<visa-resource-name>)  [unwired: 2 in, 1 out]
                n120 = call <userlib>:"Wait (ms)__ogtk.vi"("error in (no error)"=w156, "Wait on Error (FALSE)"=TRUE, "milliseconds to wait"=u32 1000) -> ("error out"=w155:errorcluster)  [unwired: 7 in, 1 out]
              }
            }
          }
        }
        n121 = local read "Stop"() -> (w132:bool)
        n122 = Not(x=w126) -> (.not. x?=w125:bool)
        n123 = Or(x=w125, y=w132) -> (x .or. y?=w127:bool)
        n124 = local write "MG.Error"(w130) -> ()
        n125 = Wait (ms)(milliseconds to wait=u32 250) -> ()  [unwired: 1 out]
      }
    }
    frame #2 {
      n126 = Set Occurrence(w207) -> ()
    }
  }
  n127 = while {
    shift-right: [w216] -> _
    shift-left: w5 -> [w222]
    shift-right: [w220] -> _
    shift-left: w5 -> [w221]
    tunnel: w7 -> [w219]
    shift-right: [w217] -> _
    shift-left: w4 -> [w218]
    shift-right: [w213] -> _
    shift-left: w5 -> [w215]
    shift-right: [w212] -> _
    shift-left: w5 -> [w214]
    tunnel: w6 -> [w211]
    shift-right: [w209] -> _
    shift-left: w4 -> [w210]
    tunnel: w3 -> [w208]
    stop <- w224 stop-if-true
    n128 = event shown="[1] <Inst.FP Public Events.MessageFromProcess>: User Event" {
      selector: w208 -> [_ _ w532 _ _ _ _ _ _ _ _ _ _ _ _ _ _ _ _ _ _ _ _ _ _ _ _ _ _ _ _]
      dyn-events: _ -> [_ _ _ _ _ _ _ _ _ _ _ _ _ _ _ _ _ _ _ _ _ _ _ _ _ _ _ _ _ _ _]
      timeout: 250 -> [_ _ _ _ _ _ _ _ _ _ _ _ _ _ _ _ _ _ _ _ _ _ _ _ _ _ _ _ _ _ _]
      tunnel: [_ _ _ TRUE _ _ _ _ _ _ _ _ _ _ _ _ _ _ _ _ _ _ _ _ _ _ _ _ _ _ _] -> w224
      tunnel: w222 -> [w225 w472 w543 w722 w758 w767 w776 w785 w797 w815 w830 w839 w845 w859 w863 w968 w984 w1000 w1017 w1022 w1042 w1052 w1067 w1074 w1082 w1090 w1101 w1118 w1134 w1157 w1162]
      tunnel: w221 -> [w228 w473 w545 w721 w757 w766 w775 w784 w796 w814 w829 w838 w843 w857 w867 w967 w985 w999 w1016 w1021 w1041 w1051 w1066 w1075 w1083 w1089 w1100 w1117 w1132 w1156 w1165]
      tunnel: [w228 w473 w544 w708 w757 w766 w775 w784 w796 w814 w829 w838 w843 w857 w867 w967 w983 w999 w1016 w1021 w1041 w1051 w1066 w1075 w1083 w1089 w1100 w1117 w1132 w1156 w1165] -> w220
      tunnel: w219 -> [_ _ w541 _ _ _ _ _ _ _ _ _ _ _ _ _ _ _ _ _ _ _ _ _ _ _ _ _ _ _ _]
      tunnel: w218 -> [w231 w474 w533 _ w756 w765 w774 w783 w793 w811 w828 w837 w851 w861 w866 w966 _ w1001 w1015 w1023 w1040 w1053 w1063 w1073 w1081 w1091 w1102 w1116 w1133 w1155 w1167]
      tunnel: [w231 w474 w535 w707 w756 w765 w774 w783 w793 w811 w828 w837 w851 w861 w866 w966 w973 w1001 w1015 w1023 w1040 w1053 w1063 w1073 w1081 w1091 w1102 w1116 w1133 w1155 w1167] -> w217
      tunnel: [w226 w472 w542 w708 w758 w767 w776 w785 w797 w815 w830 w839 w844 w858 w862 w968 w986 w1000 w1017 w1022 w1042 w1052 w1067 w1074 w1082 w1090 w1101 w1118 w1134 w1157 w1161] -> w216
      tunnel: w215 -> [w230 w476 w540 w720 w755 w764 w773 w782 w790 w808 w827 w836 w842 w856 w865 w965 w982 w998 w1013 w1020 w1039 w1050 w1065 w1077 w1084 w1088 w1099 w1114 w1131 w1153 w1164]
      tunnel: w214 -> [w229 w477 w539 w719 w754 w763 w772 w781 w789 w807 w826 w835 w841 w855 w864 w964 w980 w997 w1012 w1019 w1038 w1049 w1064 w1076 w1085 w1087 w1098 w1113 w1130 w1152 w1163]
      tunnel: [w230 w476 w538 w708 w755 w764 w773 w782 w790 w808 w827 w836 w842 w856 w865 w965 w981 w998 w1013 w1020 w1039 w1050 w1065 w1071 w1084 w1088 w1099 w1114 w1131 w1153 w1164] -> w213
      tunnel: [w229 w477 w537 w708 w754 w763 w772 w781 w789 w807 w826 w835 w841 w855 w864 w964 w979 w997 w1012 w1019 w1038 w1049 w1064 w1076 w1079 w1087 w1098 w1113 w1130 w1152 w1163] -> w212
      tunnel: w211 -> [_ _ _ w718 _ _ _ _ _ _ _ _ _ _ _ _ _ _ _ _ _ _ _ _ _ _ _ _ _ _ _]
      tunnel: w210 -> [w227 w475 w536 _ w753 w762 w771 w780 w788 w806 w825 w834 w850 w860 w869 w963 _ w988 w1014 w1018 w1028 w1045 w1062 w1070 w1078 w1086 w1097 w1115 w1129 w1154 w1166]
      tunnel: [w227 w475 w534 w707 w753 w762 w771 w780 w788 w806 w825 w834 w850 w860 w869 w963 w975 w988 w1014 w1018 w1028 w1045 w1062 w1070 w1078 w1086 w1097 w1115 w1129 w1154 w1166] -> w209
      event Timeout {
        n129 = First Call?() -> (First Call?: T/F=w232:bool)
        n130 = event-data() -> ()  [unwired: 1 in, 3 out]
        n131 = case shown="False" w232 {
          tunnel: w225 -> [w234 w415]
          tunnel: [w233 w415] -> w226
          frame False {
            n132 = stacked-sequence {
              seq-local: [w235 _ _ _] -> [_ w329 _ _]
              tunnel: w234 -> [_ _ _ w374]
              tunnel: [_ _ _ w373] -> w233
              frame #0 {
                n133 = local read "_ForceSaveData"() -> (w265:bool)
                n134 = Unbundle By Name("Logging Settings") -> ("Data Save Interval"=w272:dbl, "Save Data?"=w273:bool, "Data Plot Interval"=w264:dbl, "Plot Data?"=w274:bool)
                n135 = local read "GHS.ADC Data Array"() -> (w271:sgl[])
                n136 = local read "GHS.Status Array"() -> (w280:u32[])
                n137 = local read "PT1.Data Array"() -> (w278:dbl[])
                n138 = local read "PT2.Data Array"() -> (w263:dbl[])
                n139 = local read "MG.Data Array"() -> (w276:dbl[])
                n140 = call "Time Elapsed.vi"("Every"=w264, "Time Units"=enum16{"Minutes", "Hours", "Days"}."Minutes") -> ("Triggered?"=w268:bool)  [unwired: 1 in]
                n141 = call "Time Elapsed.vi"("Every"=w272, "Time Units"=enum16{"Minutes", "Hours", "Days"}."Minutes") -> ("Triggered?"=w269:bool)  [unwired: 1 in]
                n142 = property on="FP Error" class="Bool (strict)"() -> ("Value"=w245:bool)  [unwired: 2 in, 2 out]
                n143 = property on="MG Enabled?" class="Bool (strict)"() -> ("Value"=w248:bool)  [unwired: 2 in, 2 out]
                n144 = property on="MG Error" class="Bool (strict)"() -> ("Value"=w247:bool)  [unwired: 2 in, 2 out]
                n145 = property on="PT1.Enabled?" class="Bool (strict)"() -> ("Value"=w241:bool)  [unwired: 2 in, 2 out]
                n146 = property on="PT1 Error" class="Bool (strict)"() -> ("Value"=w249:bool)  [unwired: 2 in, 2 out]
                n147 = property on="PT2.Enabled?" class="Bool (strict)"() -> ("Value"=w243:bool)  [unwired: 2 in, 2 out]
                n148 = property on="PT2 Error" class="Bool (strict)"() -> ("Value"=w244:bool)  [unwired: 2 in, 2 out]
                n149 = Or(x=w265, y=w268) -> (x .or. y?=w266:bool)
                n150 = Or(x=w265, y=w269) -> (x .or. y?=w267:bool)
                n151 = Not(x=w245) -> (.not. x?=w239:bool)
                n152 = Not(x=w247) -> (.not. x?=w246:bool)
                n153 = Not(x=w249) -> (.not. x?=w240:bool)
                n154 = Not(x=w244) -> (.not. x?=w242:bool)
                n155 = And(x=w266, y=w274) -> (x .and. y?=w279:bool)
                n156 = And(x=w248, y=w246) -> (x .and. y?=w238:bool)
                n157 = And(x=w241, y=w240) -> (x .and. y?=w237:bool)
                n158 = And(x=w243, y=w242) -> (x .and. y?=w236:bool)
                n159 = And(x=w267, y=w273) -> (x .and. y?=w235:bool)
                n160 = case shown="True" w279 {
                  tunnel: w276 -> [_ w289]
                  tunnel: w271 -> [_ w296]
                  tunnel: w278 -> [_ w290]
                  tunnel: w263 -> [_ w284]
                  frame False {
                  }
                  frame True {
                    w283 = 1 ("Smoothing window")
                    n161 = Get Date/Time In Seconds() -> (seconds since 1Jan1904=w295:timestamp)
                    n162 = To Double Precision Float(number=w295) -> (double precision float=w294:dbl)
                    n163 = call "AppendData.vi"("Smoothing window"=w283, "Current Measurement"=w284) -> ("Data Out"=w282:sgl[][])  [unwired: 4 in]
                    n164 = call "AppendData.vi"("Smoothing window"=w283, "Current Measurement"=w296) -> ("Data Out"=w285:sgl[][])  [unwired: 4 in]
                    n165 = call "AppendData.vi"("Smoothing window"=w283, "Current Measurement"=w289) -> ("Data Out"=w286:sgl[][])  [unwired: 4 in]
                    n166 = call "AppendData.vi"("Smoothing window"=w283, "Current Measurement"=w290) -> ("Data Out"=w287:sgl[][])  [unwired: 4 in]
                    n167 = call "AppendData1.vi"("Smoothing window"=w283, "Current Measurement"=w294) -> ("Data Out"=w281:dbl[])  [unwired: 4 in]
                    n168 = call "MultiRPlot_Select1.vi"("Time"=w281, "Data In"=w285) -> ("Out Array"=→"GHS Pressures Plot":cluster{"Time":dbl[], "Value":dbl[]}[])  [unwired: 2 in]
                    n169 = call "MultiRPlot_Select1.vi"("Time"=w281, "Data In"=w286) -> ("Out Array"=→"MG Pressures Plot":cluster{"Time":dbl[], "Value":dbl[]}[])  [unwired: 2 in]
                    n170 = call "MultiRPlot_Select1.vi"("Time"=w281, "Data In"=w287) -> ("Out Array"=→"PT1 Pressures Plot":cluster{"Time":dbl[], "Value":dbl[]}[])  [unwired: 2 in]
                    n171 = call "MultiRPlot_Select1.vi"("Time"=w281, "Data In"=w282) -> ("Out Array"=→"PT2 Pressures Plot":cluster{"Time":dbl[], "Value":dbl[]}[])  [unwired: 2 in]
                  }
                }
                n172 = case shown="True" w235 {
                  tunnel: w271 -> [_ w306]
                  tunnel: w276 -> [_ w319]
                  tunnel: w280 -> [_ w318]
                  tunnel: w278 -> [_ w320]
                  tunnel: "Logging Settings" -> [_ w313]
                  tunnel: w265 -> [_ _]
                  tunnel: w263 -> [_ w301]
                  tunnel: w239 -> [_ w300]
                  tunnel: w238 -> [_ w299]
                  tunnel: w237 -> [_ w298]
                  tunnel: w236 -> [_ w297]
                  frame False {
                  }
                  frame True {
                    n173 = Unbundle By Name(w313) -> ("Filename Suffix"=w310:string, "Log Files Folder"=w312:path, "Log File Name"=w311:string, "New File Interval"=w305:u32, "Interval Units"=w304:enum16{"Minutes", "Hours", "Days"}, "Date Format"=w303:string)
                    n174 = call "Combine Data 4 logging.vi"("FP Data"=w306, "MG Data"=w319, "PT1 Data"=w320, "PT2 Data"=w301, "FP Status Bits"=w318, "Time Format String"=w303, "FP Status"=w300, "MG Status"=w299, "PT1 Status"=w298, "PT2 Status"=w297) -> ("Array"=w309:string[])  [unwired: 9 in]
                    n175 = local read "Curent Log Path"() -> (w307:path)
                    n176 = call "File Date.vi"("Cur Path"=w307) -> ("Time Stamp"=w317:timestamp)  [unwired: 4 in]
                    n177 = call "Time Elapsed time.vi"("Time Units"=w304, "Delay Time"=w305, "Time Old In"=w317) -> ("T>dT?"=w308:bool)  [unwired: 2 out]
                    n178 = case shown="True" w308 {
                      tunnel: [w322 w324] -> w315
                      tunnel: [_ w328] -> w314
                      tunnel: w312 -> [_ w327]
                      tunnel: w311 -> [_ w326]
                      tunnel: w310 -> [_ w325]
                      tunnel: w307 -> [w322 _]
                      frame False {
                      }
                      frame True {
                        n179 = call "Format header.vi"() -> ("Header string"=w323:string)  [unwired: 5 in]
                        n180 = call "GeneratePaths.vi"("Filename Suffix"=w325, "AVS_Path"=w327, "AVS_FName"=w326) -> ("Generated Log path"=w324:path)  [unwired: 11 in, 1 out]
                        n181 = Write to Text File(file (use dialog)=w324, text=w323) -> (error out=w328:errorcluster)  [unwired: 2 in, 2 out]
                      }
                    }
                    n182 = local write "_ForceSaveData"(FALSE ("ForceSave")) -> ()
                    n183 = call "Write To Spreadsheet File (string) w Error.vi"("append to file? (new file:F)"=TRUE, "error in"=w314, "1D data"=w309, "file path (dialog if empty)"=w315) -> ("new file path (Not A Path if cancelled)"=→"Curent Log Path":path)  [unwired: 6 in, 1 out]
                  }
                }
                n184 = Array To Cluster(array=w271) -> (cluster=w277:T29)
                n185 = property on="P8" class="Ring (strict)"() -> ("Value"=w275:u16)  [unwired: 2 in, 2 out]
                n186 = Index Array(array=w276, index=w275) -> (element=w250:dbl)
                n187 = Unbundle(w277) -> ("GHS.ADC Data Array[0]"=w259:sgl, "GHS.ADC Data Array[1]"=w258:sgl, "GHS.ADC Data Array[2]"=w257:sgl, "GHS.ADC Data Array[3]"=w256:sgl, "GHS.ADC Data Array[4]"=w255:sgl, "GHS.ADC Data Array[5]"=w254:sgl, "GHS.ADC Data Array[6]"=w253:sgl, "GHS.ADC Data Array[7]"=w252:sgl, "GHS.ADC Data Array[8]"=w251:sgl)
                "GHS.P6" <- w254
                "GHS.P7" <- w253
                "GHS.P2" <- w258
                "GHS.P1" <- w259
                "GHS.P3" <- w257
                "GHS.P4" <- w256
                "GHS.Flow" <- w252
                "GHS.P5" <- w255
                "GHS.PC" <- w251
                n188 = Bundle("GHS.ADC Data Array[0]"=w259, "GHS.ADC Data Array[1]"=w258, "GHS.ADC Data Array[2]"=w257, "GHS.ADC Data Array[3]"=w256, "GHS.ADC Data Array[4]"=w255, "GHS.ADC Data Array[5]"=w254, "GHS.ADC Data Array[6]"=w253, "GHS.ADC Data Array[7]"=w252, "GHS.ADC Data Array[8]"=w251, w250) -> (→"GHS.P Cluster":T30)  [unwired: 1 in]
              }
              frame #1 {
                n189 = case shown="True" w329 {
                  frame False {
                  }
                  frame True {
                    n190 = local read "GHS.ADC Data Array"() -> (w331:sgl[])
                    n191 = disable-structure shown="Disabled" {
                      frame Disabled {
                        n192 = local read "PT2.Data Array"() -> ()  [unwired: 1 out]
                      }
                      frame Enabled {
                      }
                    }
                    n193 = local read "GHS.Status Array"() -> (w335:u32[])
                    n194 = local read "MG.Data Array"() -> (w332:dbl[])
                    n195 = local read "PT1.Data Array"() -> (w333:dbl[])
                    n196 = local read "GHS.Mode"() -> (w336:u16)
                    n197 = local read "Inst.FP"() -> (w334:refnum<class "Inst.FP.lvclass">)
                    n198 = call "FP to PGSQL.vi"("Mode"=w336, "Status Array"=w335, "PT Data"=w333, "MG Data"=w332, "FP Data"=w331, "Inst.FP"=w334) -> ("Inst.FP out"=w330:refnum<class "Inst.FP.lvclass">)  [unwired: 4 in, 1 out]
                    n199 = local write "Inst.FP"(w330) -> ()
                  }
                }
              }
              frame #2 {
                # "Check if the structure is \nnot empty and only one\nof Scalar or Array controls \nis set"
                # "Set FP control value from external script/program"
                n200 = local read "_SetControl"() -> (w348:T7)
                n201 = Unbundle By Name(w348) -> ("Name"=w346:string, "Scalar"=w347:string, "Array"=w338:string[][])
                n202 = call <userlib>:"Empty 2D Array (String)__ogtk.vi"("Array"=w338) -> ("Empty Array?"=w341:bool)  [unwired: 8 in]
                n203 = Empty String/Path?(string/path=w346) -> (empty?=w342:bool)
                n204 = Empty String/Path?(string/path=w347) -> (empty?=w343:bool)
                n205 = Not(x=w342) -> (.not. x?=w344:bool)
                n206 = Not(x=w343) -> (.not. x?=w340:bool)
                n207 = Not(x=w341) -> (.not. x?=w337:bool)
                n208 = Exclusive Or(1:w337, 2:w340) -> (0:w339:bool)
                n209 = And(x=w344, y=w339) -> (x .and. y?=w345:bool)
                n210 = case shown="False" w345 {
                  tunnel: w346 -> [_ w352]
                  tunnel: w347 -> [_ w351]
                  tunnel: w338 -> [_ w350]
                  tunnel: w337 -> [_ w349]
                  frame False {
                  }
                  frame True {
                    n211 = flat-sequence {
                      tunnel: w352 -> [w356]
                      tunnel: w351 -> [w355]
                      tunnel: w350 -> [w353]
                      tunnel: w349 -> [w354]
                      frame #0 {
                        n212 = local read "VIRef"() -> (w357:T1)
                        n213 = case shown="True" w354 {
                          tunnel: w357 -> [w360 w363]
                          tunnel: w356 -> [w359 w362]
                          tunnel: w355 -> [w358 _]
                          tunnel: w353 -> [_ w361]
                          frame False {
                            n214 = call "Push2VI.vi"("New Value"=w358, "element"=w359, "VIRef"=w360) -> ()  [unwired: 8 in, 1 out]
                          }
                          frame True {
                            n215 = call "PushArray2VI.vi"("Str"=w361, "element"=w362, "VIRef"=w363) -> ()  [unwired: 8 in, 1 out]
                          }
                        }
                      }
                      frame #1 {
                        w365 = ""
                        # "Empty the cluster to flag that\nthe command is processed"
                        n216 = Bundle(w365, w365, "Array"=string[][] []) -> (→"_SetControl":cluster{string, string, "Array":string[][]})  [unwired: 1 in]
                      }
                    }
                  }
                }
              }
              frame #3 {
                n217 = local read "GHS.Error"() -> (w372:errorcluster)
                n218 = local read "MG.Error"() -> (w371:errorcluster)
                n219 = Not(x=w372) -> (.not. x?=w370:bool)
                n220 = Not(x=w371) -> (.not. x?=w369:bool)
                n221 = Compound Arithmetic op=AND(w370, w369, "Automode.Start") -> (w367:bool)
                n222 = case shown="False" w367 {
                  tunnel: w374 -> [w375 w395]
                  tunnel: [w375 w394] -> w373
                  frame False {
                    n223 = call <userlib>:"MGI Milliseconds Since Last Reset.vi"("Reset (F)"=TRUE) -> ()  [unwired: 5 in, 2 out]
                  }
                  frame True {
                    n224 = Unbundle By Name("Automode Settings") -> ("MG Channel"=w381:u16, "Threshold Pressure"=w380:dbl, "Enable Pressure Check"=w379:bool, "Delay Time"=w378:u32, "Enable Time Check"=w377:bool)
                    n225 = local read "MG.Data Array"() -> (w399:dbl[])
                    n226 = Index Array(array=w399, index=w381) -> (element=w398:dbl)
                    n227 = Not(x=w379) -> (.not. x?=w396:bool)
                    n228 = Less?(x=w398, y=w380) -> (x < y?=w397:bool)
                    n229 = Or(x=w397, y=w396) -> (x .or. y?=w384:bool)
                    "Automode.Pressure Reached?" <- w384
                    n230 = Not(x=w384) -> (.not. x?=w386:bool)
                    n231 = call <userlib>:"MGI Milliseconds Since Last Reset.vi"("Reset (F)"=w386) -> ("ms"=w393:u32)  [unwired: 5 in, 1 out]
                    n232 = Divide(x=w393, y=u32 1000) -> (x/y=w391:dbl)
                    "Automode.Delay Timer" <- w391
                    n233 = Multiply(x=w378, y=u32 60) -> (x*y=w388:u32)
                    n234 = Not(x=w377) -> (.not. x?=w389:bool)
                    n235 = Greater Or Equal?(x=w391, y=w388) -> (x >= y?=w390:bool)
                    n236 = Or(x=w390, y=w389) -> (x .or. y?=w385:bool)
                    "Automode.Time Reached?" <- w385
                    n237 = And(x=w384, y=w385) -> (x .and. y?=w383:bool)
                    "Automode.Triggered?" <- w383
                    n238 = case shown="True" w383 {
                      tunnel: w395 -> [w400 w402]
                      tunnel: [w400 w401] -> w394
                      frame False {
                      }
                      frame True {
                        # "Auto"
                        # "Start"
                        # "Reset"
                        n239 = call "BP togglekey.vi"("keynumber"=u16 10, "FrontPanel port"=w402) -> ("error out"=w414:T19, "FrontPanel port"=w409:refnum<visa-resource-name>)  [unwired: 2 in]
                        n240 = call <userlib>:"MGI Wait (U32).vi"("ms"=u32 2000, "Error In"=w414) -> ("Error Out"=w413:errorcluster)  [unwired: 5 in]
                        n241 = local write "Automode.Start"(FALSE ("EnableAutoCond")) -> ()
                        n242 = call "BP togglekey.vi"("error in"=w413, "keynumber"=u16 48, "FrontPanel port"=w409) -> ("error out"=w412:T19, "FrontPanel port"=w411:refnum<visa-resource-name>)  [unwired: 1 in]
                        n243 = call <userlib>:"MGI Wait (U32).vi"("ms"=u32 500, "Error In"=w412) -> ("Error Out"=w410:errorcluster)  [unwired: 5 in]
                        n244 = call "BP togglekey.vi"("error in"=w410, "keynumber"=u16 54, "FrontPanel port"=w411) -> ("FrontPanel port"=w401:refnum<visa-resource-name>)  [unwired: 1 in, 1 out]
                      }
                    }
                  }
                }
              }
            }
          }
          frame True {
            n245 = stacked-sequence {
              frame #0 {
                w423 = T31."Page Disabled & Grayed" ("Page Enabled State")
                w424 = u8 2 ("Disabled")
                w436 = u8 1 ("Disabled")
                w440 = u32 16777062
                w445 = u32 65382
                w444 = u32 0
                w443 = 0.1
                w442 = 2000
                w441 = 0
                n246 = property class="App"() -> ("App.Kind"=w446:T32)  [unwired: 2 in, 2 out]
                n247 = property on="Hide side panel" class="Bool (strict)"("Val(Sgnl)"=FALSE ("Value (Signaling)")) -> ()  [unwired: 2 in, 2 out]
                n248 = property on="S1" class="TabCtl (strict)"("Disabled"=w424) -> ()  [unwired: 2 in, 2 out]
                n249 = property on="S2" class="TabCtl (strict)"("Disabled"=w424) -> ()  [unwired: 2 in, 2 out]
                n250 = property on="Stop" class="Bool (strict)"("Disabled"=w424) -> ()  [unwired: 2 in, 2 out]
                n251 = property on="Error panel" class="TabCtl (strict)"("Disabled"=w424) -> ()  [unwired: 2 in, 2 out]
                n252 = property on="Main Panel Tabs" class="TabCtl (strict)"("Disabled"=w424) -> ()  [unwired: 2 in, 2 out]
                n253 = property on="Main Panel" class="TabCtl (strict)"("Disabled"=w424) -> ()  [unwired: 2 in, 2 out]
                n254 = local write "Curent Log Path"(path "") -> ()
                n255 = call <userlib>:"Current VIs Reference__ogtk.vi"() -> ("Current VI's reference"=w430:refnum<vi>)  [unwired: 5 in]
                n256 = case shown="\"Run Time System\"" w446 {
                  tunnel: [w448 w457] -> w447
                  frame "invalid app kind", Default {
                    n257 = control-ref of="This VI"() -> (w449:refnum<vi>)
                    n258 = property class="VI"(reference=w449) -> ("Hist.Revision"=w450:u32)  [unwired: 1 in, 2 out]
                    n259 = Divide(x=w450, y=1000.0 ("x")) -> (x/y=w454:dbl)
                    n260 = Number To Fractional String(use system decimal point (T)=FALSE, number=w454, precision (6)=i16 2) -> (F-format string=w455:string)  [unwired: 1 in]
                    n261 = Concatenate Strings("" ("string"), w455) -> (w448:string)
                  }
                  frame "Run Time System" {
                    n262 = call <userlib>:"MGI Get Executable Version.vi"() -> ("Version"=w457:string)  [unwired: 7 in]
                  }
                }
                "VI Version" <- w447
                n263 = call "GetFrontPanelControls.vi"("Ref to VI"=w430) -> ("VIRef"=w431:T1)  [unwired: 9 in, 1 out]
                "VIRef" <- w431
                n264 = Unbundle By Name(w431) -> ("Full Name"=→"ControlNames":string[])
                n265 = call <userlib>:"Current VI's Path__ogtk.vi"() -> ("Current VI's Path (+ Relative)"=w417:path)  [unwired: 1 in]
                n266 = property on="Side Panel" class="TabCtl (strict)"("Value"=enum32{"Main", "Settings", "Advanced"}."Settings" ("Side Panel")) -> ("Pages"=w420:refnum<vi>[])  [unwired: 2 in, 2 out]
                n267 = Path To String(path=w417) -> (string=→"_VIPath":string)
                n268 = Index Array(array=w420) -> (element #1=w421:refnum<vi>, element #3=w422:refnum<vi>)  [unwired: 3 in, 1 out]
                n269 = property class="Page"(reference=w421, "PageEnb"=w423) -> ()  [unwired: 1 in, 2 out]
                n270 = property class="Page"(reference=w422, "PageEnb"=w423) -> ()  [unwired: 1 in, 2 out]
                n271 = property on="GHS.P7" class="Slide (strict)"("Scale.Range:Minimum"=w441, "Scale.Range:Maximum"=w442, "Scale.Range:Increment"=w443) -> ()  [unwired: 2 in, 2 out]
                n272 = Initialize Array(FALSE, 64 ("dimension size")) -> (w416:bool[])
                n273 = property on="GHS.P1" class="DigNum (strict)"("Numeric Text.Text Colors:Text Color"=w444, "Numeric Text.Text Colors:BG Color"=w440) -> ()  [unwired: 2 in, 2 out]
                n274 = property on="GHS.P4" class="DigNum (strict)"("Numeric Text.Text Colors:Text Color"=w444, "Numeric Text.Text Colors:BG Color"=w445) -> ()  [unwired: 2 in, 2 out]
                n275 = property on="Start" class="Bool (strict)"("Visible"=TRUE, "Disabled"=u8 0) -> ()  [unwired: 2 in, 2 out]
                n276 = control-ref of="GHS.Layout1.LEDs"() -> (w427:refnum<vi>)
                n277 = call "FP Set Binking Controls.vi"("Cluster in"=w427, "Array of blinking states"=w416, "Array of relais states"=w416) -> ()  [unwired: 13 in]
                n278 = property on="Hardware Settings" class="Clust (strict)"("Disabled"=u8 0) -> ()  [unwired: 2 in, 2 out]
                n279 = property on="GHS.P2" class="DigNum (strict)"("Numeric Text.Text Colors:Text Color"=w444, "Numeric Text.Text Colors:BG Color"=w440) -> ()  [unwired: 2 in, 2 out]
                n280 = property on="GHS.P5" class="DigNum (strict)"("Numeric Text.Text Colors:Text Color"=w444, "Numeric Text.Text Colors:BG Color"=w445) -> ()  [unwired: 2 in, 2 out]
                n281 = property on="GHS.P6" class="Slide (strict)"("Scale.Range:Minimum"=w441, "Scale.Range:Maximum"=w442, "Scale.Range:Increment"=w443) -> ()  [unwired: 2 in, 2 out]
                n282 = control-ref of="GHS.Layout2.LEDs"() -> (w428:refnum<vi>)
                n283 = call "FP Set Binking Controls.vi"("Cluster in"=w428, "Array of blinking states"=w416, "Array of relais states"=w416) -> ()  [unwired: 13 in]
                n284 = property on="GHS.P3" class="DigNum (strict)"("Numeric Text.Text Colors:Text Color"=w444, "Numeric Text.Text Colors:BG Color"=w440) -> ()  [unwired: 2 in, 2 out]
                n285 = property on="GHS.Flow" class="DigNum (strict)"("Numeric Text.Text Colors:Text Color"=w444, "Numeric Text.Text Colors:BG Color"=w445) -> ()  [unwired: 2 in, 2 out]
                n286 = property on="GHS.Panel ID" class="Str"("Text.Text Colors:Text Color"=u32 13311) -> ()  [unwired: 2 in, 2 out]
                n287 = property on="GHS.Layout1.Buttons" class="Clust"("Disabled"=w436) -> ()  [unwired: 2 in, 2 out]
                n288 = property on="GHS.Layout2.Buttons" class="Clust"("Disabled"=w436) -> ()  [unwired: 2 in, 2 out]
                n289 = local write "Automode.Start"(FALSE ("EnableAutoCond")) -> ()
              }
              frame #1 {
                # "First load the settings from the old location then \nfrom the new one. This way the program will \"transfer\" \nthe settings to the new config file after the upgrade"
                n290 = call <userlib>:"Create Dir if Non-Existant__ogtk.vi"("Directory Path"=path "C:/LC Data/Configuration/FP" ("Relative path (.)")) -> ("dup Directory Path"=w460:path)  [unwired: 8 in, 2 out]
                n291 = call <userlib>:"Build Path - Traditional__ogtk.vi"("name or relative path"="FP config.ini", "base path"=w460) -> ("appended path"=w458:path)
                n292 = control-ref of="Hardware Settings"() -> (w470:refnum<vi>)
                n293 = control-ref of="GHS.ADC scaling"() -> (w467:refnum<vi>)
                n294 = control-ref of="Logging Settings"() -> (w466:refnum<vi>)
                n295 = call <userlib>:"Current VIs Parent Directory__ogtk.vi"("Relative path (.)"=path "config.ini") -> ("Parent Directory (+ Relative)"=w468:path)  [unwired: 4 in]
                n296 = Build Array(w470, w467, w466) -> (w463:refnum<vi>[])
                n297 = call "Save Load Settings to File by Ref with path.vi"("Array of Cluster References"=w463, "Action"=enum8{"Load", "Save"}."Load", "Configuration file"=w468) -> ("error out"=w464:errorcluster)  [unwired: 6 in]
                n298 = call <userlib>:"MGI Clear Error.vi"("Error In"=w464) -> ("Error Out"=w465:errorcluster)  [unwired: 6 in]
                n299 = call "Save Load Settings to File by Ref with path.vi"("Array of Cluster References"=w463, "Action"=enum8{"Load", "Save"}."Load", "error in (no error)"=w465, "Configuration file"=w458) -> ()  [unwired: 5 in, 1 out]
              }
            }
          }
        }
      }
      event User Event {
        n300 = event-data() -> ("Message.Command"=w481:string, "Message.Data"=w479:variant, "Message.ID"=w478:string)  [unwired: 1 in]
        n301 = local read "Inst.FP"() -> (w483:refnum<class "Inst.FP.lvclass">)
        n302 = case shown="\"Push Button\"" w481 {
          tunnel: w483 -> [w486 w499]
          tunnel: [w486 w499] -> w482
          tunnel: ["ACK" "ACK"] -> w480
          tunnel: w479 -> [_ w496]
          frame Default {
          }
          frame "Push Button" {
            n303 = property on="GHS.Layout1.Buttons" class="Clust"() -> ("Value"=w492:variant)  [unwired: 2 in, 2 out]
            n304 = Variant To Data(type="", Variant=w496) -> (data=w489:string, error out=w497:errorcluster)  [unwired: 1 in]
            n305 = call "From JSON Text.vim"("Data Type and Default Value"=T27 {"Button"=enum."Start"} ("Set State"), "error in (no error)"=w497, "JSON"=w489) -> ("Data out"=w495:T27)  [unwired: 7 in, 1 out]
            n306 = Variant To Data(type=T4 {"baux2"=FALSE, "bBypass"=FALSE, "b15"=FALSE, "b16"=FALSE, "NC 0"=FALSE, "baux1"=FALSE, "b4"=FALSE, "NC 1"=FALSE, "b5"=FALSE, "breset"=FALSE, "NC 2"=FALSE, "b9"=FALSE, "b14"=FALSE, "NC 3"=FALSE, "b13"=FALSE, "bledtest"=FALSE, "NC 4"=FALSE, "b12"=FALSE, "b10"=FALSE, "NC 5"=FALSE, "b11"=FALSE, "bA0"=FALSE, "NC 9"=FALSE, "b7"=FALSE, "bS3"=FALSE, "NC 12"=FALSE, "b6"=FALSE, "b17"=FALSE, "NC 13"=FALSE, "b8"=FALSE, "b1"=FALSE, "NC 14"=FALSE, "bS2"=FALSE, "b3"=FALSE, "NC 15"=FALSE, "b2"=FALSE, "b0"=FALSE, "NC 16"=FALSE, "bS1"=FALSE, "bA9"=FALSE, "NC 17"=FALSE, "bA8"=FALSE, "bA2"=FALSE, "NC 6"=FALSE, "bs5"=FALSE, "bA10"=FALSE, "NC 7"=FALSE, "bstart"=FALSE, "bA5"=FALSE, "NC 8"=FALSE, "bA7"=FALSE, "bA1"=FALSE, "NC 10"=FALSE, "bauto"=FALSE, "bA4"=FALSE, "NC 11"=FALSE, "bA6"=FALSE, "bS4"=FALSE, "NC 18"=FALSE, "bA3"=FALSE, "b3he"=FALSE, "b4he"=FALSE, "bnorm"=FALSE, "brecov"=FALSE} ("GHS.Layout1.Buttons"), Variant=w492) -> (data=w491:T4)  [unwired: 1 in, 1 out]
            n307 = Unbundle(w495) -> ("Button"=w494:T28)
            n308 = case shown="\"Reset\"" w494 {
              tunnel: w491 -> [w502 w506 w510 w514 w518 w522 w526 w530]
              tunnel: [w503 w507 w511 w515 w519 w523 w527 w531] -> w493
              frame "Start", Default {
                n309 = Unbundle By Name(w502) -> ("bstart"=w501:bool)
                n310 = Not(x=w501) -> (.not. x?=w500:bool)
                n311 = Bundle By Name(cluster=w502, "bstart"=w500) -> (w503:T4)
              }
              frame "3He" {
                n312 = Unbundle By Name(w506) -> ("b3he"=w505:bool)
                n313 = Not(x=w505) -> (.not. x?=w504:bool)
                n314 = Bundle By Name(cluster=w506, "b3he"=w504) -> (w507:T4)
              }
              frame "4He" {
                n315 = Unbundle By Name(w510) -> ("b4he"=w509:bool)
                n316 = Not(x=w509) -> (.not. x?=w508:bool)
                n317 = Bundle By Name(cluster=w510, "b4he"=w508) -> (w511:T4)
              }
              frame "Normal" {
                n318 = Unbundle By Name(w514) -> ("bnorm"=w513:bool)
                n319 = Not(x=w513) -> (.not. x?=w512:bool)
                n320 = Bundle By Name(cluster=w514, "bnorm"=w512) -> (w515:T4)
              }
              frame "Recovery" {
                n321 = Unbundle By Name(w518) -> ("brecov"=w517:bool)
                n322 = Not(x=w517) -> (.not. x?=w516:bool)
                n323 = Bundle By Name(cluster=w518, "brecov"=w516) -> (w519:T4)
              }
              frame "Auto" {
                n324 = Unbundle By Name(w522) -> ("bauto"=w521:bool)
                n325 = Not(x=w521) -> (.not. x?=w520:bool)
                n326 = Bundle By Name(cluster=w522, "bauto"=w520) -> (w523:T4)
              }
              frame "LED Test" {
                n327 = Unbundle By Name(w526) -> ("bledtest"=w525:bool)
                n328 = Not(x=w525) -> (.not. x?=w524:bool)
                n329 = Bundle By Name(cluster=w526, "bledtest"=w524) -> (w527:T4)
              }
              frame "Reset" {
                n330 = Unbundle By Name(w530) -> ("breset"=w529:bool)
                n331 = Not(x=w529) -> (.not. x?=w528:bool)
                n332 = Bundle By Name(cluster=w530, "breset"=w528) -> (w531:T4)
              }
            }
            n333 = property on="GHS.Layout1.Buttons" class="Clust"("Val(Sgnl)"=w493) -> ()  [unwired: 2 in, 2 out]
          }
        }
        n334 = call <userlib>:"Instrument.MessageToProcess.vi"("ID"=w478, "Command"=w480, "Instrument"=w482) -> ("Instrument out"=w484:refnum<class "Inst.FP.lvclass">)  [unwired: 7 in, 1 out]
        n335 = local write "Inst.FP"(w484) -> ()
      }
      event "Start": Value Change {
        n336 = event-data() -> ()  [unwired: 1 in, 6 out]
        n337 = stacked-sequence {
          tunnel: w545 -> [_ w595 _ _ _ _ _]
          tunnel: [_ w594 _ _ _ _ _] -> w544
          tunnel: w543 -> [w560 _ _ _ _ _ _]
          tunnel: [w547 _ _ _ _ _ _] -> w542
          tunnel: w541 -> [_ _ _ _ _ _ w706]
          tunnel: w540 -> [_ _ _ w667 _ _ _]
          tunnel: w539 -> [_ _ _ w666 _ _ _]
          tunnel: [_ _ _ w664 _ _ _] -> w538
          tunnel: [_ _ _ w665 _ _ _] -> w537
          tunnel: w533 -> [_ _ _ _ _ _ _]
          tunnel: w536 -> [_ _ _ _ _ _ _]
          tunnel: [_ _ w622 _ _ _ _] -> w535
          tunnel: [_ _ w626 _ _ _ _] -> w534
          tunnel: w532 -> [_ _ _ _ _ w701 _]
          frame #0 {
            n338 = call "Stop Display Busy AE.vi"("Action"=enum16{"Write", "Read"}."Write", "Error In"=T19 {"error"=FALSE, "code"=0, "source"=""} ("error in"), "Stop?"=FALSE) -> ("Error Out"=w548:errorcluster)  [unwired: 7 in, 1 out]
            n339 = property on="GHS Bauds" class="DigNum (strict)"() -> ("Value"=w559:u32)  [unwired: 2 in, 2 out]
            n340 = call "FP-Scan ports.vi"("Error in"=w548, "baud rate"=w559, "RS232 port"=w560) -> ("Error out"=w551:errorcluster, "ID string"=w557:string, "VISA Refnum out"=w558:refnum<visa-resource-name>)  [unwired: 5 in, 1 out]
            "GHS.Panel ID" <- w557
            n341 = call "Stop Display Busy AE.vi"("Action"=enum16{"Write", "Read"}."Write", "Error In"=w551, "Stop?"=TRUE) -> ("Error Out"=w550:errorcluster)  [unwired: 7 in, 1 out]
            n342 = call "Get GHS version and type.vi"("ID string"=w557, "error in (no error)"=w550) -> ("Panel Version"=w565:bool, "System Type"=w564:bool, "error out"=w561:errorcluster)  [unwired: 4 in]
            n343 = call "Display Busy.vi"("error in (no error)"=w548, "Title"="Trying to connect to the Front Panel") -> ()  [unwired: 8 in, 2 out]
            n344 = Boolean To (0,1)(Boolean=w565) -> (0, 1=w546:i16)
            n345 = Boolean To (0,1)(Boolean=w564) -> (0, 1=w563:i16)
            n346 = property on="GHS Layout Panel" class="TabCtl (strict)"("Value"=w546) -> ()  [unwired: 2 in, 2 out]
            n347 = property on="GHS.Layout" class="Enum (strict)"("Value"=w546) -> ()  [unwired: 2 in, 2 out]
            n348 = property on="GHS.System Type" class="RadioBtnsControl (strict)"("Val(Sgnl)"=w563) -> ()  [unwired: 2 in, 2 out]
            n349 = call "BP query settings.vi"("error in"=w561, "FrontPanel port"=w558) -> ("error out"=w562:T19, "array of 4 x 16 bit unsigned"=w572:u16[], "FrontPanel port"=w573:refnum<visa-resource-name>)  [unwired: 2 in, 1 out]
            "GHS.Error" <- w562
            n350 = call "BP query P5.vi"("error in"=w562, "FrontPanel port"=w573) -> ("error out"=w586:T19, "array of 2 x 16 bit unsigned"=w591:u16[], "FrontPanel port"=w592:refnum<visa-resource-name>)  [unwired: 2 in, 1 out]
            n351 = Array To Cluster(array=w572) -> (cluster=w571:T33)
            n352 = Array To Cluster(array=w591) -> (cluster=w584:T34)
            n353 = call "Disable on error.vi"("error out"=w586) -> ("Numeric"=w587:i16)
            n354 = property on="GHS.P6&7 Limits" class="Clust (strict)"("Value"=w571) -> ()  [unwired: 2 in, 2 out]
            n355 = call "BP query NCP5.vi"("error in"=w562, "FrontPanel port"=w592) -> ("error out"=w589:T19, "array of 3 x 16 bit unsigned"=w590:u16[], "FrontPanel port"=w583:refnum<visa-resource-name>)  [unwired: 2 in, 1 out]
            n356 = property on="GHS.P5 Settings" class="Clust (strict)"("Value"=w584, "Disabled"=w587) -> ()  [unwired: 2 in, 2 out]
            n357 = Array To Cluster(array=w590) -> (cluster=w585:T35)
            n358 = call "Disable on error.vi"("error out"=w589) -> ("Numeric"=w588:i16)
            n359 = call "BP query NCP5B.vi"("error in"=w562, "FrontPanel port"=w583) -> ("error out"=w580:T19, "array of 3 x 16 bit unsigned"=w581:u16[], "FrontPanel port"=w582:refnum<visa-resource-name>)  [unwired: 2 in, 1 out]
            n360 = property on="GHS.NCP5 Settings" class="Clust (strict)"("Value"=w585, "Disabled"=w588) -> ()  [unwired: 2 in, 2 out]
            n361 = Array To Cluster(array=w581) -> (cluster=w578:cluster{"array of 3 x 16 bit unsigned[0]":u16})
            n362 = property on="GHS.P6&7 Settings" class="Clust (strict)"("Value"=w571) -> ()  [unwired: 2 in, 2 out]
            n363 = call "Disable on error.vi"("error out"=w580) -> ("Numeric"=w579:i16)
            n364 = call "BP Query REC.vi"("error in"=w562, "FrontPanel port"=w582) -> ("error out"=w576:T19, "array of 3 x 16 bit unsigned"=w577:u16[], "FrontPanel port"=w570:refnum<visa-resource-name>)  [unwired: 2 in, 1 out]
            n365 = property on="GHS.P5 limits" class="Clust (strict)"("Value"=w584) -> ()  [unwired: 2 in, 2 out]
            n366 = property on="GHS.NCP5B Settings" class="Clust (strict)"("Value"=w578, "Disabled"=w579) -> ()  [unwired: 2 in, 2 out]
            n367 = Array To Cluster(array=w577) -> (cluster=w574:T35)
            n368 = call "Disable on error.vi"("error out"=w576) -> ("Numeric"=w575:i16)
            n369 = call "BP Query Turbo.vi"("error in"=w562, "FrontPanel port"=w570) -> ("error out"=w568:T19, "array of 3 x 16 bit unsigned"=w567:u16[], "FrontPanel port"=w547:refnum<visa-resource-name>)  [unwired: 2 in, 1 out]
            "_GHSPort" <- w547
            n370 = property on="GHS.REC Settings" class="Clust (strict)"("Value"=w574, "Disabled"=w575) -> ()  [unwired: 2 in, 2 out]
            n371 = property on="GHS.NCP5 limits" class="Clust (strict)"("Value"=w585) -> ()  [unwired: 2 in, 2 out]
            n372 = Array To Cluster(array=w567) -> (cluster=w566:cluster{"array of 3 x 16 bit unsigned[0]":u16})
            n373 = call "Disable on error.vi"("error out"=w568) -> ("Numeric"=w569:i16)
            n374 = property on="GHS.S1&2 Settings" class="Clust (strict)"("Value"=w566, "Disabled"=w569) -> ()  [unwired: 2 in, 2 out]
            n375 = property on="GHS.NCP5B limits" class="Clust (strict)"("Value"=w578) -> ()  [unwired: 2 in, 2 out]
            n376 = property on="GHS.REC limits" class="Clust (strict)"("Value"=w574) -> ()  [unwired: 2 in, 2 out]
            n377 = property on="GHS Port" class="VISAName"("Value"=w547) -> ()  [unwired: 2 in, 2 out]
            n378 = property on="GHS.S1&2 limits" class="Clust (strict)"("Value"=w566) -> ()  [unwired: 2 in, 2 out]
          }
          frame #1 {
            w597 = T19 {"error"=FALSE, "code"=0, "source"=""}  # No error
            n379 = property on="MG Enabled?" class="Bool (strict)"() -> ("Value"=w596:bool)  [unwired: 2 in, 2 out]
            n380 = case shown="True" w596 {
              tunnel: [w600 w617] -> w593
              tunnel: [w598 w601] -> w594
              tunnel: w597 -> [w600 w607]
              tunnel: [FALSE TRUE] -> _
              tunnel: w595 -> [w598 w612]
              frame False {
                # "MaxiGauge not connected"
              }
              frame True {
                n381 = call "Stop Display Busy AE.vi"("Action"=enum16{"Write", "Read"}."Write", "Error In"=w607, "Stop?"=FALSE) -> ("Error Out"=w602:errorcluster)  [unwired: 7 in, 1 out]
                n382 = call "MG- Scan ports.vi"("Error in"=w602, "RS232 port"=w612) -> ("Error out"=w604:errorcluster, "ID string"=→"MG.ID String":string, "VISA Refnum out"=w611:refnum<visa-resource-name>)  [unwired: 6 in, 1 out]
                n383 = call "Stop Display Busy AE.vi"("Action"=enum16{"Write", "Read"}."Write", "Error In"=w604, "Stop?"=TRUE) -> ()  [unwired: 7 in, 2 out]
                n384 = call "Display Busy.vi"("error in (no error)"=w602, "Title"="Trying to connect to the MaxiGauge") -> ()  [unwired: 8 in, 2 out]
                n385 = call "MG Get Channels Labels.vi"("MaxiGauge port"=w611) -> ("Array"=w615:string[], "MaxiGauge port"=w601:refnum<visa-resource-name>, "error out"=w617:errorcluster)  [unwired: 1 in]
                "_MGPort" <- w601
                n386 = Array To Cluster(array=w615) -> (cluster=→"MG.Channel Names":T36)
                n387 = for {
                  tunnel: w615 -> [w620] mode=indexing
                  i -> [w621]
                  n388 = property on="MG Pressures Plot" class="XYGraph (strict)"("Active Plot"=w621, "Plot.Plot Name"=w620, "Plot.Visible?"=TRUE ("Plot.Visible")) -> ()  [unwired: 2 in, 2 out]
                }
                n389 = Search 1D Array(1D array=w615, element="STIL") -> (index of element=w613:i32)  [unwired: 1 in]
                n390 = property on="MG P8 Channel" class="Ring (strict)"("Value"=w613) -> ()  [unwired: 2 in, 2 out]
                n391 = property on="MG Port" class="VISAName"("Value"=w601) -> ()  [unwired: 2 in, 2 out]
              }
            }
            "MG.Error" <- w593
          }
          frame #2 {
            n392 = property on="PT1 port \nnumber" class="VISAName"() -> ("Value"=w625:refnum<visa-resource-name>)  [unwired: 2 in, 2 out]
            n393 = property on="PT1.Enabled?" class="Bool (strict)"() -> ("Value"=w631:bool)  [unwired: 2 in, 2 out]
            n394 = case shown="True" w631 {
              tunnel: w625 -> [_ w663]
              tunnel: [u16 0 ("Port Number out") w662] -> w622
              tunnel: [errorcluster {"status"=FALSE, "code"=0, "source"=""} ("Error out") w654] -> w630
              tunnel: [refnum<visa-resource-name> refnum ("VISA Refnum out") w651] -> w623
              frame False {
              }
              frame True {
                n395 = call "Stop Display Busy AE.vi"("Action"=enum16{"Write", "Read"}."Write", "Stop?"=FALSE) -> ("Error Out"=w652:errorcluster)  [unwired: 8 in, 1 out]
                n396 = property on="PT1 Bauds" class="DigNum (strict)"() -> ("Value"=w661:u32)  [unwired: 2 in, 2 out]
                n397 = property on="PT1 Address" class="DigNum (strict)"() -> ("Value"=w660:u8)  [unwired: 2 in, 2 out]
                n398 = call "PT-Scan ports.vi"("Error in"=w652, "PT Address"=w660, "Baud rate"=w661, "RS232 port"=w663) -> ("Error out"=w655:errorcluster, "Port Number out"=w662:u16, "serial Port out"=w651:refnum<visa-resource-name>)  [unwired: 3 in, 2 out]
                n399 = call "Display Busy.vi"("error in (no error)"=w652, "Title"="Trying to connect to PulseTube1") -> ()  [unwired: 8 in, 2 out]
                n400 = property on="PT1 Port" class="VISAName"("Value"=w651) -> ()  [unwired: 2 in, 2 out]
                n401 = call "Stop Display Busy AE.vi"("Action"=enum16{"Write", "Read"}."Write", "Error In"=w655, "Stop?"=TRUE) -> ("Error Out"=w654:errorcluster)  [unwired: 7 in, 1 out]
              }
            }
            "PT1.Error" <- w630
            "_PT1Port" <- w622
            n402 = property on="PT2 port \nnumber" class="VISAName"() -> ("Value"=w624:refnum<visa-resource-name>)  [unwired: 2 in, 2 out]
            n403 = property on="PT2.Enabled?" class="Bool (strict)"() -> ("Value"=w628:bool)  [unwired: 2 in, 2 out]
            n404 = Build Array(w623) -> (w629:refnum<visa-resource-name>[])
            n405 = case shown="True" w628 {
              tunnel: w624 -> [_ w647]
              tunnel: [u16 0 ("Port Number out") w646] -> w626
              tunnel: [errorcluster {"status"=FALSE, "code"=0, "source"=""} ("Error out") w635] -> w627
              tunnel: w629 -> [_ w643]
              frame False {
              }
              frame True {
                n406 = call "Stop Display Busy AE.vi"("Action"=enum16{"Write", "Read"}."Write", "Stop?"=FALSE) -> ("Error Out"=w639:errorcluster)  [unwired: 8 in, 1 out]
                n407 = property on="PT2 Bauds" class="DigNum (strict)"() -> ("Value"=w645:u32)  [unwired: 2 in, 2 out]
                n408 = property on="PT2 Address" class="DigNum (strict)"() -> ("Value"=w644:u8)  [unwired: 2 in, 2 out]
                n409 = call "PT-Scan ports.vi"("RS232 ports to skip"=w643, "Error in"=w639, "PT Address"=w644, "Baud rate"=w645, "RS232 port"=w647) -> ("Error out"=w636:errorcluster, "Port Number out"=w646:u16, "serial Port out"=w634:refnum<visa-resource-name>)  [unwired: 2 in, 2 out]
                n410 = call "Display Busy.vi"("error in (no error)"=w639, "Title"="Trying to connect to PulseTube2") -> ()  [unwired: 8 in, 2 out]
                n411 = property on="PT2 Port" class="VISAName"("Value"=w634) -> ()  [unwired: 2 in, 2 out]
                n412 = call "Stop Display Busy AE.vi"("Action"=enum16{"Write", "Read"}."Write", "Error In"=w636, "Stop?"=TRUE) -> ("Error Out"=w635:errorcluster)  [unwired: 7 in, 1 out]
              }
            }
            "PT2.Error" <- w627
            "_PT2Port" <- w626
          }
          frame #3 {
            n413 = disable-structure shown="Enabled" {
              disable-tunnel: w667 -> [w673 w681]
              disable-tunnel: w666 -> [w672 w680]
              disable-tunnel: [w671 w680] -> w665
              disable-tunnel: [w668 w681] -> w664
              frame Disabled {
                n414 = property on="S2 Enabled?" class="Bool (strict)"() -> ("Value"=w669:bool)  [unwired: 2 in, 2 out]
                n415 = property on="S1 Enabled?" class="Bool (strict)"() -> ("Value"=w670:bool)  [unwired: 2 in, 2 out]
                n416 = case shown="False" w670 {
                  tunnel: w673 -> [w677 w679]
                  tunnel: [w677 w678] -> w668
                  frame False {
                  }
                  frame True {
                    n417 = call "PV Initialize.vi"("VISA session in"=w679) -> ("VISA session out"=w678:refnum<visa-resource-name>)  [unwired: 9 in, 1 out]
                  }
                }
                n418 = case shown="True" w669 {
                  tunnel: w672 -> [w674 w676]
                  tunnel: [w674 w675] -> w671
                  frame False {
                  }
                  frame True {
                    n419 = call "PV Initialize.vi"("VISA session in"=w676) -> ("VISA session out"=w675:refnum<visa-resource-name>)  [unwired: 9 in, 1 out]
                  }
                }
              }
              frame Enabled {
              }
            }
          }
          frame #4 {
            w683 = T31."Page Enabled" ("Page Enabled State")
            w688 = u8 0 ("Disabled")
            w691 = u8 0 ("Disabled")
            n420 = property on="Hardware Settings" class="Clust (strict)"("Disabled"=u8 2) -> ()  [unwired: 2 in, 2 out]
            n421 = property on="GHS.Layout1.Buttons" class="Clust"("Disabled"=w691) -> ()  [unwired: 2 in, 2 out]
            n422 = property on="GHS.Layout2.Buttons" class="Clust"("Disabled"=w691) -> ()  [unwired: 2 in, 2 out]
            n423 = local write "Start"(FALSE ("Start")) -> ()
            n424 = property on="Main Panel Tabs" class="TabCtl (strict)"("Disabled"=w688) -> ()  [unwired: 2 in, 2 out]
            n425 = property on="Main Panel" class="TabCtl (strict)"("Disabled"=w688) -> ()  [unwired: 2 in, 2 out]
            n426 = property on="Stop" class="Bool (strict)"("Disabled"=w688) -> ()  [unwired: 2 in, 2 out]
            n427 = property on="Error panel" class="TabCtl (strict)"("Disabled"=w688) -> ()  [unwired: 2 in, 2 out]
            n428 = property on="Side Panel" class="TabCtl (strict)"("Value"=enum32{"Main", "Settings", "Advanced"}."Main" ("Side Panel")) -> ("Pages"=w685:refnum<vi>[])  [unwired: 2 in, 2 out]
            n429 = Index Array(array=w685) -> (element #1=w686:refnum<vi>, element #2=w682:refnum<vi>, element #3=w687:refnum<vi>)  [unwired: 3 in]
            n430 = property class="Page"(reference=w686, "PageEnb"=w683) -> ()  [unwired: 1 in, 2 out]
            n431 = property class="Page"(reference=w682, "PageEnb"=w683) -> ()  [unwired: 1 in, 2 out]
            n432 = property class="Page"(reference=w687, "PageEnb"=w683) -> ()  [unwired: 1 in, 2 out]
          }
          frame #5 {
            # "This frame will run after the Start button is pressed. The start button will initiate the hardware enumeration\nand the software will query the GHS hardware/EPROM for the system type (Wet/CF, New/Old layout, etc)."
            # "replace MessageFromProcess refnum"
            n433 = call "Stop Display Busy AE.vi"("Action"=enum16{"Write", "Read"}."Write", "Stop?"=FALSE) -> ("Error Out"=w693:errorcluster)  [unwired: 8 in, 1 out]
            n434 = local read "GHS.System Type"() -> (w694:enum32{"Wet", "CF"})
            n435 = local read "Inst.FP"() -> (w700:refnum<class "Inst.FP.lvclass">)
            n436 = call "Display Busy.vi"("error in (no error)"=w693, "Title"="Starting Inst.FP SMO") -> ()  [unwired: 8 in, 2 out]
            n437 = call "Inst.FP.Create.vi"("error in (no error)"=w693, "FP Type"=w694, "Inst.FP in"=w700) -> ("error out"=w692:errorcluster, "Inst.FP Public Events"=w702:T18, "Inst.FP out"=w703:refnum<class "Inst.FP.lvclass">)  [unwired: 6 in]
            n438 = local write "Inst.FP"(w703) -> ()
            n439 = call "Stop Display Busy AE.vi"("Action"=enum16{"Write", "Read"}."Write", "Error In"=w692, "Stop?"=TRUE) -> ()  [unwired: 7 in, 2 out]
            n440 = register-events(reference=w701, w702) -> ()  [unwired: 1 in, 2 out]
          }
          frame #6 {
            n441 = Set Occurrence(w706) -> ()
            n442 = property on="Start" class="Bool (strict)"("Visible"=TRUE, "Disabled"=u8 2) -> ()  [unwired: 2 in, 2 out]
          }
        }
      }
      event "Stop": Value Change {
        w707 = u16 0 ("Port Number out")
        w708 = refnum<visa-resource-name> refnum ("PT port")
        n443 = event-data() -> ()  [unwired: 1 in, 6 out]
        n444 = call "Stop Display Busy AE.vi"("Action"=enum16{"Write", "Read"}."Write", "Stop?"=FALSE) -> ("Error Out"=w711:errorcluster)  [unwired: 8 in, 1 out]
        n445 = call "Display Busy.vi"("error in (no error)"=w711, "Title"="Stopping...") -> ()  [unwired: 8 in, 2 out]
        n446 = flat-sequence {
          tunnel: w718 -> [w725]
          tunnel: [w724] -> w713
          tunnel: w711 -> [w724]
          tunnel: w722 -> [w729]
          tunnel: w721 -> [w727]
          tunnel: w720 -> [w728]
          tunnel: w719 -> [w730]
          tunnel: [w726] -> w714
          tunnel: w713 -> [w726]
          tunnel: [w732] -> w715
          tunnel: w714 -> [w731]
          tunnel: w715 -> [w744]
          tunnel: [w743] -> w710
          tunnel: w710 -> [w749]
          tunnel: [w749] -> w709
          tunnel: w709 -> [_]
          frame #0 {
            n447 = Wait on Occurrence(2:w725) -> ()  [unwired: 2 in, 1 out]
          }
          frame #1 {
            n448 = VISA Close(VISA resource name=w729) -> ()  [unwired: 1 in, 1 out]
            n449 = VISA Close(VISA resource name=w727) -> ()  [unwired: 1 in, 1 out]
            n450 = VISA Close(VISA resource name=w728) -> ()  [unwired: 1 in, 1 out]
            n451 = VISA Close(VISA resource name=w730) -> ()  [unwired: 1 in, 1 out]
          }
          frame #2 {
            n452 = local read "Inst.FP"() -> (w735:refnum<class "Inst.FP.lvclass">)
            n453 = control-ref of="Hardware Settings"() -> (w740:refnum<vi>)
            n454 = control-ref of="GHS.ADC scaling"() -> (w738:refnum<vi>)
            n455 = control-ref of="Logging Settings"() -> (w737:refnum<vi>)
            n456 = call <vilib>:"Stop.vi"("error in (no error)"=w731, "SMO"=w735) -> ("error out"=w733:errorcluster, "SMO out"=w734:refnum<class "Inst.FP.lvclass">)  [unwired: 8 in]
            n457 = property on="Start" class="Bool (strict)"("Visible"=TRUE) -> ()  [unwired: 2 in, 2 out]
            n458 = call <vilib>:"Destroy.vi"("error in (no error)"=w733, "SMO"=w734) -> ("error out"=w732:errorcluster)  [unwired: 9 in]
            n459 = Build Array(w740, w738, w737) -> (w741:refnum<vi>[])
            n460 = call "Save Load Settings to File by Ref with path.vi"("Array of Cluster References"=w741, "Action"=enum8{"Load", "Save"}."Save", "Configuration file"=path "C:/LC Data/Configuration/FP/FP config.ini" ("Relative path (.)")) -> ()  [unwired: 6 in, 1 out]
          }
          frame #3 {
            n461 = call "Stop Display Busy AE.vi"("Action"=enum16{"Write", "Read"}."Write", "Error In"=w744, "Stop?"=TRUE) -> ("Error Out"=w743:errorcluster)  [unwired: 7 in, 1 out]
            n462 = property on="Stop" class="Bool (strict)"("Value"=FALSE ("stop")) -> ()  [unwired: 2 in, 2 out]
          }
          frame #4 {
            n463 = Wait (ms)(milliseconds to wait=u32 500) -> ()  [unwired: 1 out]
          }
          frame #5 {
            n464 = Stop(stop? (T)=TRUE) -> ()
          }
        }
      }
      event "PT1.Start": Value Change {
        w759 = u16 54529 items=["Compressor START"=54529, "Compressor STOP"=50584, "Error Code"=26020, "Reset Max/Min"=54235] ("Command")
        n465 = event-data() -> ()  [unwired: 1 in, 6 out]
        n466 = property on="PT1 Address" class="DigNum (strict)"() -> ("Value"=w752:u8)  [unwired: 2 in, 2 out]
        n467 = property on="PT1 Bauds" class="DigNum (strict)"() -> ("Value"=w751:u32)  [unwired: 2 in, 2 out]
        n468 = call "PT Send Command.vi"("PT1 port"=w756, "PT Address"=w752, "PT Bauds"=w751, "Command"=w759) -> ()  [unwired: 1 in, 2 out]
      }
      event "PT2.Start": Value Change {
        w768 = u16 54529 items=["Compressor START"=54529, "Compressor STOP"=50584, "Error Code"=26020, "Reset Max/Min"=54235] ("Command")
        n469 = event-data() -> ()  [unwired: 1 in, 6 out]
        n470 = property on="PT2 Address" class="DigNum (strict)"() -> ("Value"=w761:u8)  [unwired: 2 in, 2 out]
        n471 = property on="PT2 Bauds" class="DigNum (strict)"() -> ("Value"=w760:u32)  [unwired: 2 in, 2 out]
        n472 = call "PT Send Command.vi"("PT1 port"=w762, "PT Address"=w761, "PT Bauds"=w760, "Command"=w768) -> ()  [unwired: 1 in, 2 out]
      }
      event "PT1.Stop": Value Change {
        w777 = u16 50584 items=["Compressor START"=54529, "Compressor STOP"=50584, "Error Code"=26020, "Reset Max/Min"=54235] ("Command")
        n473 = event-data() -> ()  [unwired: 1 in, 1 out]
        n474 = property on="PT1 Address" class="DigNum (strict)"() -> ("Value"=w770:u8)  [unwired: 2 in, 2 out]
        n475 = property on="PT1 Bauds" class="DigNum (strict)"() -> ("Value"=w769:u32)  [unwired: 2 in, 2 out]
        n476 = call "PT Send Command.vi"("PT1 port"=w774, "PT Address"=w770, "PT Bauds"=w769, "Command"=w777) -> ()  [unwired: 1 in, 2 out]
      }
      event "PT2.Stop": Value Change {
        w786 = u16 50584 items=["Compressor START"=54529, "Compressor STOP"=50584, "Error Code"=26020, "Reset Max/Min"=54235] ("Command")
        n477 = event-data() -> ()  [unwired: 1 in, 1 out]
        n478 = property on="PT2 Address" class="DigNum (strict)"() -> ("Value"=w779:u8)  [unwired: 2 in, 2 out]
        n479 = property on="PT2 Bauds" class="DigNum (strict)"() -> ("Value"=w778:u32)  [unwired: 2 in, 2 out]
        n480 = call "PT Send Command.vi"("PT1 port"=w780, "PT Address"=w779, "PT Bauds"=w778, "Command"=w786) -> ()  [unwired: 1 in, 2 out]
      }
      event "PT1.Error Code": Value Change {
        n481 = event-data() -> ("OldVal"=w795:i32, "NewVal"=w791:i32)  [unwired: 1 in]
        n482 = Not Equal?(x=w795, y=w791) -> (x != y?=w794:bool)
        n483 = global read "ErrCodeStatusLkup.vi" "Error code/name/description Firmware V1.5"() -> (w792:string)
        n484 = Pick Line(multi-line string=w792, line index=w791) -> (output string=w787:string)  [unwired: 1 in]
        "PT1.Error Text" <- w787
        n485 = case shown="True" w794 {
          tunnel: w791 -> [_ w801]
          tunnel: w787 -> [_ w798]
          frame False {
          }
          frame True {
            n486 = Format Date/Time String() -> (date/time string=w799:string)  [unwired: 3 in]
            n487 = Number To Decimal String(number=w801) -> (decimal integer string=w800:string)  [unwired: 1 in]
            n488 = Build Array(w799, w800, w798) -> (w802:string[])
            n489 = feedback #1() -> (w803:string[][])  [unwired: 1 in]
            "PT1.Error Log" <- w803
            n490 = Build Array (concatenate)(w803, w802) -> (w804:string[][])
            n491 = feedback-in #1(w804) -> ()
          }
        }
      }
      event "PT2.Error Code": Value Change {
        n492 = event-data() -> ("OldVal"=w813:i32, "NewVal"=w809:i32)  [unwired: 1 in]
        n493 = Not Equal?(x=w813, y=w809) -> (x != y?=w812:bool)
        n494 = global read "ErrCodeStatusLkup.vi" "Error code/name/description Firmware V1.5"() -> (w810:string)
        n495 = Pick Line(multi-line string=w810, line index=w809) -> (output string=w805:string)  [unwired: 1 in]
        "PT2.Error Text" <- w805
        n496 = case shown="True" w812 {
          tunnel: w809 -> [_ w819]
          tunnel: w805 -> [_ w816]
          frame False {
          }
          frame True {
            n497 = Format Date/Time String() -> (date/time string=w817:string)  [unwired: 3 in]
            n498 = Number To Decimal String(number=w819) -> (decimal integer string=w818:string)  [unwired: 1 in]
            n499 = Build Array(w817, w818, w816) -> (w820:string[])
            n500 = feedback #2() -> (w821:string[][])  [unwired: 1 in]
            "PT2.Error Log" <- w821
            n501 = Build Array (concatenate)(w821, w820) -> (w822:string[][])
            n502 = feedback-in #2(w822) -> ()
          }
        }
      }
      event "PT1.ResetValues": Value Change {
        w831 = u16 54235 items=["Compressor START"=54529, "Compressor STOP"=50584, "Error Code"=26020, "Reset Max/Min"=54235] ("Command")
        n503 = event-data() -> ()  [unwired: 1 in, 1 out]
        n504 = property on="PT1 Address" class="DigNum (strict)"() -> ("Value"=w824:u8)  [unwired: 2 in, 2 out]
        n505 = property on="PT1 Bauds" class="DigNum (strict)"() -> ("Value"=w823:u32)  [unwired: 2 in, 2 out]
        n506 = call "PT Send Command.vi"("PT1 port"=w828, "PT Address"=w824, "PT Bauds"=w823, "Command"=w831) -> ()  [unwired: 1 in, 2 out]
      }
      event "PT2.ResetValues": Value Change {
        w840 = u16 54235 items=["Compressor START"=54529, "Compressor STOP"=50584, "Error Code"=26020, "Reset Max/Min"=54235] ("Command")
        n507 = event-data() -> ()  [unwired: 1 in, 1 out]
        n508 = property on="PT2 Address" class="DigNum (strict)"() -> ("Value"=w833:u8)  [unwired: 2 in, 2 out]
        n509 = property on="PT2 Bauds" class="DigNum (strict)"() -> ("Value"=w832:u32)  [unwired: 2 in, 2 out]
        n510 = call "PT Send Command.vi"("PT1 port"=w834, "PT Address"=w833, "PT Bauds"=w832, "Command"=w840) -> ()  [unwired: 1 in, 2 out]
      }
      event "GHS.Layout2.Buttons", "GHS.Layout1.Buttons": Value Change {
        n511 = event-data() -> ("NewVal"=w849:T4)  [unwired: 1 in, 5 out]
        n512 = Cluster To Array(cluster=w849) -> (array=w848:bool[])
        n513 = while {
          tunnel: w848 -> [w853] mode=indexing
          tunnel: [w852] -> w847
          i -> [w852]
          stop <- w853 stop-if-true
        }
        n514 = Increment(x=w847) -> (x+1=w846:i32)
        n515 = call "BP togglekey.vi"("keynumber"=w846, "FrontPanel port"=w845) -> ("FrontPanel port"=w844:refnum<visa-resource-name>)  [unwired: 2 in, 1 out]
      }
      event "GHS.Button": Value Change {
        n516 = event-data() -> ()  [unwired: 1 in, 6 out]
        n517 = call "BP togglekey.vi"("keynumber"="GHS.Button", "FrontPanel port"=w859) -> ("FrontPanel port"=w858:refnum<visa-resource-name>)  [unwired: 2 in, 1 out]
      }
      event "GHS.Set Values": Value Change {
        n518 = event-data() -> ("OldVal"=w868:bool)  [unwired: 1 in, 5 out]
        n519 = property on="GHS.Set Values" class="Bool (strict)"("Value"=w868) -> ()  [unwired: 2 in, 2 out]
        n520 = stacked-sequence {
          tunnel: w863 -> [w874 w888 w903 w921 w936 w951]
          tunnel: [w870 _ _ _ _ _] -> w862
          frame #0 {
            n521 = local read "GHS.P6&7 Settings"() -> (w873:T13)
            n522 = local read "GHS.P6&7 Limits"() -> (w872:T13)
            n523 = Not Equal?(x=w873, y=w872) -> (x != y?=w871:bool)
            n524 = case shown="True" w871 {
              tunnel: w874 -> [w876 w883]
              tunnel: [w876 w882] -> w870
              frame False {
                n525 = control-ref of="GHS.P6&7 Settings"() -> (w875:refnum<vi>)
                n526 = call "FP check parameters error.vi"("Clust Refnum"=w875) -> ()  [unwired: 6 in, 1 out]
              }
              frame True {
                n527 = control-ref of="GHS.P6&7 Settings"() -> (w879:refnum<vi>)
                n528 = call "BP Set Config.vi"("GHS Settings"="GHS.P6&7 Settings", "FrontPanel port"=w883) -> ("error out"=w881:T19, "FrontPanel port"=w887:refnum<visa-resource-name>)  [unwired: 2 in]
                n529 = call "FP check parameters error.vi"("error in"=w881, "Clust Refnum"=w879) -> ("error out"=w880:errorcluster)  [unwired: 5 in]
                n530 = call "BP query settings.vi"("error in"=w880, "FrontPanel port"=w887) -> ("error out"=w878:T19, "array of 4 x 16 bit unsigned"=w885:u16[], "BP response"=→"GHS.Response":string, "FrontPanel port"=w882:refnum<visa-resource-name>)  [unwired: 2 in]
                n531 = Array To Cluster(array=w885) -> (cluster=→"GHS.P6&7 Limits":T33)
                n532 = local write "GHS.Error"(w878) -> ()
              }
            }
          }
          frame #1 {
            n533 = local read "GHS.P5 Settings"() -> (w890:cluster{"P6 low":u16, "P6 high":u16})
            n534 = local read "GHS.P5 limits"() -> (w891:cluster{"P5 C1":u16, "P5 C2":u16})
            n535 = Not Equal?(x=w890, y=w891) -> (x != y?=w889:bool)
            n536 = case shown="True" w889 {
              tunnel: w888 -> [_ w898]
              frame False {
                n537 = control-ref of="GHS.P5 Settings"() -> (w892:refnum<vi>)
                n538 = call "FP check parameters error.vi"("Clust Refnum"=w892) -> ()  [unwired: 6 in, 1 out]
              }
              frame True {
                n539 = control-ref of="GHS.P5 Settings"() -> (w895:refnum<vi>)
                n540 = call "BP Set P5.vi"("P5 Settings"="GHS.P5 Settings", "FrontPanel port in"=w898) -> ("error out"=w902:errorcluster, "FrontPanel port out"=w901:refnum<visa-resource-name>)  [unwired: 2 in]
                n541 = call "FP check parameters error.vi"("error in"=w902, "Clust Refnum"=w895) -> ("error out"=w896:errorcluster)  [unwired: 5 in]
                n542 = call "BP query P5.vi"("error in"=w896, "FrontPanel port"=w901) -> ("error out"=w894:T19, "array of 2 x 16 bit unsigned"=w900:u16[], "BP response"=w893:string)  [unwired: 2 in, 1 out]
                n543 = Array To Cluster(array=w900) -> (cluster=→"GHS.P5 limits":T34)
                n544 = local write "GHS.Response"(w893) -> ()
                n545 = local write "GHS.Error"(w894) -> ()
              }
            }
          }
          frame #2 {
            n546 = local read "GHS.NCP5 Settings"() -> (w905:T10)
            n547 = local read "GHS.NCP5 limits"() -> (w906:T12)
            n548 = Not Equal?(x=w905, y=w906) -> (x != y?=w904:bool)
            n549 = case shown="True" w904 {
              tunnel: w903 -> [_ w913]
              frame False {
                n550 = control-ref of="GHS.NCP5 Settings"() -> (w907:refnum<vi>)
                n551 = call "FP check parameters error.vi"("Clust Refnum"=w907) -> ()  [unwired: 6 in, 1 out]
              }
              frame True {
                n552 = control-ref of="GHS.NCP5 Settings"() -> (w910:refnum<vi>)
                n553 = call "BP Set NCP5.vi"("NCP5 Settings"="GHS.NCP5 Settings", "FrontPanel port in"=w913) -> ("error out"=w912:errorcluster, "FrontPanel port out"=w917:refnum<visa-resource-name>)  [unwired: 2 in]
                n554 = call "FP check parameters error.vi"("error in"=w912, "Clust Refnum"=w910) -> ("error out"=w911:errorcluster)  [unwired: 5 in]
                n555 = call "BP query NCP5.vi"("error in"=w911, "FrontPanel port"=w917) -> ("error out"=w909:T19, "array of 3 x 16 bit unsigned"=w915:u16[], "BP response"=w908:string)  [unwired: 2 in, 1 out]
                n556 = local write "GHS.Response"(w908) -> ()
                n557 = local write "GHS.Error"(w909) -> ()
                n558 = Array To Cluster(array=w915) -> (cluster=→"GHS.NCP5 limits":T35)
              }
            }
          }
          frame #3 {
            n559 = local read "GHS.NCP5B Settings"() -> (w918:cluster{"P6 low":u16})
            n560 = local read "GHS.NCP5B limits"() -> (w919:cluster{"P5 NC4":u16})
            n561 = Not Equal?(x=w918, y=w919) -> (x != y?=w920:bool)
            n562 = case shown="True" w920 {
              tunnel: w921 -> [_ w928]
              frame False {
                n563 = control-ref of="GHS.NCP5B Settings"() -> (w922:refnum<vi>)
                n564 = call "FP check parameters error.vi"("Clust Refnum"=w922) -> ()  [unwired: 6 in, 1 out]
              }
              frame True {
                n565 = control-ref of="GHS.NCP5B Settings"() -> (w925:refnum<vi>)
                n566 = call "BP Set NCP5B.vi"("NCP5B"="GHS.NCP5B Settings", "FrontPanel port in"=w928) -> ("error out"=w927:errorcluster, "FrontPanel port out"=w929:refnum<visa-resource-name>)  [unwired: 2 in]
                n567 = call "FP check parameters error.vi"("error in"=w927, "Clust Refnum"=w925) -> ("error out"=w926:errorcluster)  [unwired: 5 in]
                n568 = call "BP query NCP5B.vi"("error in"=w926, "FrontPanel port"=w929) -> ("error out"=w924:T19, "array of 3 x 16 bit unsigned"=w930:u16[], "BP response"=w923:string)  [unwired: 2 in, 1 out]
                n569 = local write "GHS.Response"(w923) -> ()
                n570 = Array To Cluster(array=w930) -> (cluster=→"GHS.NCP5B limits":cluster{"array of 3 x 16 bit unsigned[0]":u16})
                n571 = local write "GHS.Error"(w924) -> ()
              }
            }
          }
          frame #4 {
            n572 = local read "GHS.REC Settings"() -> (w934:T10)
            n573 = local read "GHS.REC limits"() -> (w935:T11)
            n574 = Not Equal?(x=w934, y=w935) -> (x != y?=w933:bool)
            n575 = case shown="True" w933 {
              tunnel: w936 -> [_ w943]
              frame False {
                n576 = control-ref of="GHS.REC Settings"() -> (w937:refnum<vi>)
                n577 = call "FP check parameters error.vi"("Clust Refnum"=w937) -> ()  [unwired: 6 in, 1 out]
              }
              frame True {
                n578 = control-ref of="GHS.REC Settings"() -> (w940:refnum<vi>)
                n579 = call "BP Set REC.vi"("NCP5 Settings"="GHS.REC Settings", "FrontPanel port in"=w943) -> ("error out"=w942:errorcluster, "FrontPanel port out"=w944:refnum<visa-resource-name>)  [unwired: 2 in]
                n580 = call "FP check parameters error.vi"("error in"=w942, "Clust Refnum"=w940) -> ("error out"=w941:errorcluster)  [unwired: 5 in]
                n581 = call "BP Query REC.vi"("error in"=w941, "FrontPanel port"=w944) -> ("error out"=w939:T19, "array of 3 x 16 bit unsigned"=w946:u16[], "BP response"=w938:string)  [unwired: 2 in, 1 out]
                n582 = local write "GHS.Response"(w938) -> ()
                n583 = Array To Cluster(array=w946) -> (cluster=→"GHS.REC limits":T35)
                n584 = local write "GHS.Error"(w939) -> ()
              }
            }
          }
          frame #5 {
            n585 = local read "GHS.S1&2 Settings"() -> (w948:cluster{"Enum":enum16{"OFF", "ON"}})
            n586 = local read "GHS.S1&2 limits"() -> (w949:cluster{"S1&S2":enum16{"OFF", "ON"}})
            n587 = Not Equal?(x=w948, y=w949) -> (x != y?=w950:bool)
            n588 = case shown="True" w950 {
              tunnel: w951 -> [_ w960]
              frame False {
                n589 = control-ref of="GHS.S1&2 Settings"() -> (w952:refnum<vi>)
                n590 = call "FP check parameters error.vi"("Clust Refnum"=w952) -> ()  [unwired: 6 in, 1 out]
              }
              frame True {
                n591 = control-ref of="GHS.S1&2 Settings"() -> (w955:refnum<vi>)
                n592 = call "BP Set Turbo.vi"("S1&2 Settings"="GHS.S1&2 Settings", "FrontPanel port in"=w960) -> ("error out"=w957:errorcluster, "FrontPanel port out"=w961:refnum<visa-resource-name>)  [unwired: 2 in]
                n593 = call "FP check parameters error.vi"("error in"=w957, "Clust Refnum"=w955) -> ("error out"=w956:errorcluster)  [unwired: 5 in]
                n594 = call "BP Query Turbo.vi"("error in"=w956, "FrontPanel port"=w961) -> ("error out"=w954:T19, "array of 3 x 16 bit unsigned"=w962:u16[], "BP response"=w953:string)  [unwired: 2 in, 1 out]
                n595 = local write "GHS.Response"(w953) -> ()
                n596 = Array To Cluster(array=w962) -> (cluster=→"GHS.S1&2 limits":cluster{"array of 3 x 16 bit unsigned[0]":u16})
                n597 = local write "GHS.Error"(w954) -> ()
              }
            }
          }
        }
      }
      event "Logging Settings.Plot Data?": Value Change {
        n598 = event-data() -> ("NewVal"=w969:bool)  [unwired: 1 in, 5 out]
        n599 = property on="Main Panel Tabs" class="TabCtl (strict)"() -> ("Pages"=w972:refnum<vi>[])  [unwired: 2 in, 2 out]
        n600 = Index Array(array=w972, index=2) -> (element=w970:refnum<vi>)
        n601 = property class="Page"(reference=w970, "PageVis"=w969) -> ()  [unwired: 1 in, 2 out]
      }
      event "Hardware Settings": Value Change {
        n602 = event-data() -> ()  [unwired: 1 in, 6 out]
        n603 = VISA Close(VISA resource name=w984) -> ()  [unwired: 1 in, 1 out]
        n604 = VISA Close(VISA resource name=w985) -> ()  [unwired: 1 in, 1 out]
        n605 = VISA Close(VISA resource name=w982) -> ()  [unwired: 1 in, 1 out]
        n606 = VISA Close(VISA resource name=w980) -> ()  [unwired: 1 in, 1 out]
        n607 = Unbundle By Name("Hardware Settings") -> ("PT1 Port"=w974:refnum<visa-resource-name>, "PT2 Port"=w976:refnum<visa-resource-name>, "GHS Port"=w986:refnum<visa-resource-name>, "MG Port"=w983:refnum<visa-resource-name>, "S1 port"=w981:refnum<visa-resource-name>, "S2 port"=w979:refnum<visa-resource-name>)
        n608 = call "VISA to RS232 Port Nr.vi"("VISA Resource Name"=w974) -> ("Port Number"=w978:u8)
        n609 = call "VISA to RS232 Port Nr.vi"("VISA Resource Name"=w976) -> ("Port Number"=w977:u8)
        n610 = Increment(x=w978) -> (x+1=w973:u8)
        n611 = Increment(x=w977) -> (x+1=w975:u8)
      }
      event "GHS.System Type": Value Change {
        n612 = event-data() -> ("NewVal"=w991:enum32{"Wet", "CF"})  [unwired: 1 in, 5 out]
        n613 = case shown="\"Wet\"" w991 {
          tunnel: ["COMPRESSOR" ("Label.Text") "AUX 2" ("Label.Text")] -> w996
          tunnel: [TRUE ("Visible") FALSE ("Visible")] -> w992
          tunnel: ["From\nProbe" ("Text.Text") "From\nDewar" ("Text.Text")] -> w990
          tunnel: ["From\nOVC" ("Text.Text") "From\n1K pot" ("Text.Text")] -> w989
          frame "CF", Default {
          }
          frame "Wet" {
          }
        }
        n614 = property on="Main Panel Tabs" class="TabCtl (strict)"() -> ("Pages"=w995:refnum<vi>[])  [unwired: 2 in, 2 out]
        n615 = property on="COMPR/AUX 2" class="Bool (strict)"("Caption.Text"=w996) -> ()  [unwired: 2 in, 2 out]
        n616 = property on="GHS.Layout1.Label2" class="Str"("Text.Text"=w990) -> ()  [unwired: 2 in, 2 out]
        n617 = property on="GHS.Layout1.Label1" class="Str"("Text.Text"=w989) -> ()  [unwired: 2 in, 2 out]
        n618 = Index Array(array=w995, index=1) -> (element=w993:refnum<vi>)
        n619 = property on="BYPASS" class="Bool (strict)"("Visible"=w992) -> ()  [unwired: 2 in, 2 out]
        n620 = property on="PT STATUS" class="Bool (strict)"("Visible"=w992) -> ()  [unwired: 2 in, 2 out]
        n621 = property class="Page"(reference=w993, "PageVis"=w992) -> ()  [unwired: 1 in, 2 out]
        n622 = property on="GHS.Layout2.Label2" class="Str"("Text.Text"=w990) -> ()  [unwired: 2 in, 2 out]
        n623 = property on="GHS.Layout2.Label1" class="Str"("Text.Text"=w989) -> ()  [unwired: 2 in, 2 out]
      }
      event "GHS.Layout": Value Change {
        n624 = event-data() -> ("NewVal"=w1010:enum32{"Layout1", "Layout2"})  [unwired: 1 in, 5 out]
        n625 = To Unsigned Long Integer(number=w1010) -> (unsigned 32bit integer=w1011:u32)
        n626 = property on="GHS Layout Panel" class="TabCtl (strict)"("Value"=w1011) -> ()  [unwired: 2 in, 2 out]
      }
      event "GHS.Status Array": Value Change {
        n627 = event-data() -> ("OldVal"=w1026:u32[], "NewVal"=w1025:u32[])  [unwired: 1 in, 4 out]
        n628 = Not Equal?(x=w1026, y=w1025) -> (x != y?=w1024:bool)
        n629 = case shown="True" w1024 {
          frame False {
          }
          frame True {
            "_ForceSaveData" <- TRUE ("ForceSave")
          }
        }
      }
      event "GHS Pressures Plot", "MG Pressures Plot": Shortcut Menu Activation? {
        w1032 = string[] ["Log Y"] ("item names")
        w1044 = string[] ["Autoscale XY"] ("item names")
        n630 = event-data() -> ("MenuRef"=w1030:refnum<k9>, "CtlRef"=w1029:refnum<vi>)  [unwired: 1 in]
        n631 = Insert Menu Items(4:10, 7:w1044, 8:w1044, 9:w1030) -> (3:w1031:refnum<k9>)  [unwired: 2 in, 2 out]
        n632 = property class="XYGraph (strict)"(reference=w1029) -> ("YScale.Mapping Mode"=w1035:u8)  [unwired: 1 in, 2 out]
        n633 = Insert Menu Items(4:13, 7:w1032, 8:w1032, 9:w1031) -> (3:w1034:refnum<k9>)  [unwired: 2 in, 2 out]
        n634 = Not Equal To 0?(x=w1035) -> (x != 0?=w1036:bool)
        n635 = Set Menu Item Info(6:w1036, 7:"Log Y", 11:w1034) -> ()  [unwired: 4 in, 2 out]
        n636 = event-data() -> ()  [unwired: 2 in, 1 out]
      }
      event "GHS Pressures Plot", "MG Pressures Plot": Shortcut Menu Selection (User) {
        n637 = event-data() -> ("CtlRef"=w1048:refnum<vi>, "ItemTag"=w1054:string)  [unwired: 1 in]
        n638 = Type Cast(type=refnum<vi> refnum ("R-Plot 0"), x=w1048) -> (*(type *) &x=w1047:refnum<vi>)
        n639 = case shown="\"Log Y\"" w1054 {
          tunnel: w1047 -> [_ w1055 w1057]
          frame Default {
          }
          frame "Autoscale XY" {
            w1056 = u8 2 ("X Scale.Scale Fit")
            n640 = property class="XYGraph (strict)"(reference=w1055, "XScale.ScaleFit"=w1056, "YScale.ScaleFit"=w1056) -> ()  [unwired: 1 in, 2 out]
          }
          frame "Log Y" {
            n641 = property class="XYGraph (strict)"(reference=w1057) -> (reference out=w1058:refnum<vi>, "YScale.Mapping Mode"=w1059:u8)  [unwired: 1 in, 1 out]
            n642 = Equal To 0?(x=w1059) -> (x = 0?=w1060:bool)
            n643 = Boolean To (0,1)(Boolean=w1060) -> (0, 1=w1061:i16)
            n644 = property class="XYGraph (strict)"(reference=w1058, "YScale.Mapping Mode"=w1061) -> ()  [unwired: 1 in, 2 out]
          }
        }
      }
      event "GHS Pressures Plot", "MG Pressures Plot": Scale Range Change {
        w1069 = u8 0 ("X Scale.Scale Fit")
        n645 = event-data() -> ("CtlRef"=w1068:refnum<vi>)  [unwired: 1 in, 7 out]
        n646 = property class="XYGraph (strict)"(reference=w1068, "XScale.ScaleFit"=w1069, "YScale.ScaleFit"=w1069) -> ()  [unwired: 1 in, 2 out]
      }
      event "S1:Reset Error": Value Change {
        n647 = event-data() -> ()  [unwired: 1 in, 6 out]
        n648 = property on="Device address S1" class="DigNum (strict)"() -> ("Value"=w1072:u8)  [unwired: 2 in, 2 out]
        n649 = call "PV Error Reset.vi"("Adress of unit"=w1072, "VISA session"=w1077) -> ("VISA resource out"=w1071:refnum<visa-resource-name>)  [unwired: 8 in, 1 out]
      }
      event "S2:Reset Error": Value Change {
        n650 = event-data() -> ()  [unwired: 1 in, 6 out]
        n651 = property on="Device address S2" class="DigNum (strict)"() -> ("Value"=w1080:u8)  [unwired: 2 in, 2 out]
        n652 = call "PV Error Reset.vi"("Adress of unit"=w1080, "VISA session"=w1085) -> ("VISA resource out"=w1079:refnum<visa-resource-name>)  [unwired: 8 in, 1 out]
      }
      event "Hardware Settings.S1 Enabled?": Value Change {
        n653 = event-data() -> ("NewVal"=w1096:bool)  [unwired: 1 in, 5 out]
        n654 = Not(x=w1096) -> (.not. x?=w1095:bool)
        n655 = Boolean To (0,1)(Boolean=w1095) -> (0, 1=w1094:i16)
        n656 = Multiply(x=i16 2, y=w1094) -> (x*y=w1092:i16)
        n657 = property on="S1" class="TabCtl (strict)"("Disabled"=w1092) -> ()  [unwired: 2 in, 2 out]
      }
      event "Hardware Settings.S2 Enabled?": Value Change {
        n658 = event-data() -> ("NewVal"=w1104:bool)  [unwired: 1 in, 5 out]
        n659 = Not(x=w1104) -> (.not. x?=w1107:bool)
        n660 = Boolean To (0,1)(Boolean=w1107) -> (0, 1=w1106:i16)
        n661 = Multiply(x=i16 2, y=w1106) -> (x*y=w1103:i16)
        n662 = property on="S2" class="TabCtl (strict)"("Disabled"=w1103) -> ()  [unwired: 2 in, 2 out]
      }
      event "Hardware Settings.PT1.Enabled?", "Hardware Settings.PT2.Enabled?": Value Change {
        n663 = event-data() -> ()  [unwired: 1 in, 6 out]
        n664 = property on="PT1.Enabled?" class="Bool (strict)"() -> ("Value"=w1109:bool)  [unwired: 2 in, 2 out]
        n665 = property on="PT2.Enabled?" class="Bool (strict)"() -> ("Value"=w1108:bool)  [unwired: 2 in, 2 out]
        n666 = property on="Main Panel Tabs" class="TabCtl (strict)"() -> ("Pages"=w1112:refnum<vi>[])  [unwired: 2 in, 2 out]
        n667 = Or(x=w1109, y=w1108) -> (x .or. y?=w1110:bool)
        n668 = Index Array(array=w1112) -> (element #2=w1111:refnum<vi>)  [unwired: 2 in, 1 out]
        n669 = property class="Page"(reference=w1111, "PageVis"=w1110) -> ()  [unwired: 1 in, 2 out]
      }
      event "Hide Side Panel": Value Change {
        w1120 = T37 {"Horizontal"=0, "Vertical"=-24} ("Origin")
        w1119 = T37 {"Horizontal"=0, "Vertical"=0} ("Origin")
        # "right"
        # "left"
        n670 = event-data() -> ("NewVal"=w1135:bool)  [unwired: 1 in, 5 out]
        n671 = case shown="False" w1135 {
          frame True {
            n672 = property class="VI"() -> ("Front Panel.PanelBounds"=w1136:T38)  [unwired: 2 in, 2 out]
            n673 = Unbundle By Name(w1136) -> ("Left"=w1142:i16, "Top"=w1139:i16)
            n674 = Add(x=i16 955 ("right"), y=w1142) -> (x+y=w1141:i16)
            n675 = Add(x=w1139, y=i16 730) -> (x+y=w1137:i16)
            n676 = Bundle By Name(cluster=w1136, "Right"=w1141, "Bottom"=w1137) -> (w1143:T38)
            n677 = property class="VI"("Front Panel.PanelBounds"=w1143) -> ()  [unwired: 2 in, 2 out]
          }
          frame False {
            n678 = property class="VI"() -> ("Front Panel.PanelBounds"=w1144:T38)  [unwired: 2 in, 2 out]
            n679 = Unbundle By Name(w1144) -> ("Left"=w1150:i16, "Top"=w1147:i16)
            n680 = Add(x=i16 1259 ("right"), y=w1150) -> (x+y=w1149:i16)
            n681 = Add(x=w1147, y=i16 730) -> (x+y=w1145:i16)
            n682 = Bundle By Name(cluster=w1144, "Right"=w1149, "Bottom"=w1145) -> (w1151:T38)
            n683 = property class="VI"("Front Panel.PanelBounds"=w1151) -> ()  [unwired: 2 in, 2 out]
          }
        }
        n684 = control-ref of="Pane 2"() -> (w1128:refnum<vi>)
        n685 = property class="Pane"(reference=w1128, "Origin"=w1119) -> ()  [unwired: 1 in, 2 out]
        n686 = Unbundle By Name(w1119) -> ("Horizontal"=w1123:i16, "Vertical"=w1122:i16)
        n687 = control-ref of="Pane 3"() -> (w1127:refnum<vi>)
        n688 = property class="Pane"(reference=w1127, "Origin"=w1120) -> ()  [unwired: 1 in, 2 out]
        n689 = Unbundle By Name(w1120) -> ("Horizontal"=w1125:i16, "Vertical"=w1124:i16)
        n690 = Format Into String(format string="Left:\nH %d\nV %d\nRight:\nH %d\nV%d", w1125, w1124, w1123, w1122) -> (resulting string=→"String":string)  [unwired: 2 in, 1 out]
      }
      event "GHS Pressures Plot", "MG Pressures Plot": Plot Attribute Change {
        n691 = event-data() -> ()  [unwired: 1 in, 8 out]
        n692 = local write "_ForceSaveData"(TRUE ("ForceSave")) -> ()
      }
      event "GHS.Send Command": Value Change {
        n693 = event-data() -> ()  [unwired: 1 in, 6 out]
        n694 = call "BP Send Command.vi"("String"="GHS.Command to Send", "FrontPanel port in"=w1162) -> ("string after ack"=→"GHS.Command Response":string, "FrontPanel port out"=w1161:refnum<visa-resource-name>)  [unwired: 1 in, 1 out]
      }
    }
  }
